vi "Fiber Auto Collimation Apex.vi"() -> ()   [LabVIEW 2018]
doc: "This is the actual top-level VI. It is called \"Apex\" instead of \"Main\" because it has the command handling in it but it's not the main front panel, so it's not a \"Main\" VI in the usual sense."
uses:
  State data/Permission levels.ctl
  <userlib>/Recipe/Station Config/Station config.lvclass
  C:/Program Files (x86)/National Instruments/LabVIEW 2018/user.lib/Recipe/nLight Recipe/nLight Recipe.lvclass
  State data/Fiber Auto Collimation state data.lvclass
  Panels/Fiber Auto Collimation panel.lvclass
  <instrlib>/nLight Instruments/Beam Profiler/Beam Profiler.lvclass
  <instrlib>/nLight Instruments/Motion Controller/Specific Models/Thorlabs Kinesis/Thorlabs motion.lvclass
  <instrlib>/nLight Instruments/Motion Controller/Motion Controller.lvclass
  <instrlib>/nLight Instruments/Motion Controller/Specific Models/Thorlabs Kinesis/Monitor/Thorlabs Monitor.lvclass
  <userlib>/nEQdb/Test Data classes/Test Data.lvclass
  <userlib>/nEQdb/Test Data classes/Standard Laser Data/Standard Laser Data.lvclass
  C:/Program Files (x86)/National Instruments/LabVIEW 2018/user.lib/nEQdb/Test Data classes/Test Data.lvclass
  <instrlib>/nLight Instruments/Beam Profiler/Specific Models/BeamView/BeamView.lvclass
  State data/Fiber Auto Collimation state data.lvclass/Fiber Auto Collimation state data.ctl
  State data/Station status.ctl
  State data/String keys.ctl
  <userlib>/Recipe/Station Config/Station config.lvclass/Station config.ctl
  <instrlib>/nLight Instruments/nLight Instrument/nLight Instrument.lvclass
  <userlib>/nLight Tidbits/Logging/Controls/Logging type choice.ctl
  Error handling/Model error handling data.ctl
  Queueing/Model queue data.ctl
  <userlib>/Recipe/nLight Recipe/Recipe problem handling method.ctl
  <userlib>/Recipe/WebService/Base URI for MOM recipe management.ctl
  Queueing/Selective queue clearing methods.ctl
  <userlib>/nLight Tidbits/Logging/Controls/Logging setup FGV options.ctl
  <userlib>/nLight Tidbits/Logging/Controls/Logging to options.ctl
  State data/Tracked state data.ctl
  <userlib>/Recipe/Station Config/Bulk startup options.ctl
  State data/Instrument list.ctl
  Panels/Main panel/Fiber Auto Collimation main panel.lvclass
  <instrlib>/nLight Instruments/Motion Controller/Axis index.ctl
  Panels/Configuration panel/Fiber Auto Collimation configuration panel.lvclass
  C:/LabVIEW Code/Fiber Auto Collimation/Source/Panels/Fiber Auto Collimation panel.lvclass
  State data/Boolean keys.ctl
  State data/Integer keys.ctl
  State data/Float keys.ctl
  <userlib>/Recipe/Test Recipe classes/Test Recipe.lvclass
  c91f844a-f770-4daa-9f60-3301e0a5f322.vi
  b3d8b4fd-21fb-468c-bd3f-db48a488eb2a.vi
  efb2ec2a-33ad-4281-ad92-67e4d6b6ec68.vi
  ae384ee7-eaaf-47a0-aaff-5ccb6f93d8a1.vi
  a18a64c1-f4c2-4f15-aef6-8607d0dc9e34.vi
  997a605e-7b1f-4adb-a0e7-d1eb57c4fb87.vi
  c0a0718e-5dff-4a87-91f2-0d7809bf613b.vi
  82acb594-edb5-4f8a-8fca-e4c401c4994d.vi
  54d7c561-c5ff-4c4f-ad18-53407e4e607b.vi
  2cd3d775-6c45-4b39-8171-6f7e11c70f95.vi
  8a1b4983-7c71-4597-b233-a9b8e1038a8c.vi
  eb02f1ea-705f-4cce-9035-a9f8b34ca533.vi
  828f032b-9937-4802-b0e2-0a19cdc0ac1c.vi
  76d71b13-37a6-4cc4-9b9a-5e2ce6ce3de4.vi
  d3521ccb-280c-4964-8afe-59c39be19f88.vi
  12af3aa9-4c13-45d6-86bd-f229a8c437ee.vi
  <userlib>/nLight Tidbits/Misc/Convert True to Enabled.vi
  997a605e-7b1f-4adb-a0e7-d1eb57c4fb87.vi/a2caca50-23ab-4663-8cbd-eebdf5a4aabe.vi
  c0a0718e-5dff-4a87-91f2-0d7809bf613b.vi/9db3fc61-2e1c-4885-9405-90c6bc597e16.vi
  References/Obtain control updates queue.vi
  Misc SubVIs/Get control name.vi
  <vilib>/Utility/Data Type/Get Type Information.vi
  <userlib>/nLight Error Handling/Log any errors.vi
  <userlib>/nLight Error Handling/Replace string to enum conversion error.vi
  <vilib>/Platform/browser.llb/Open URL in Default Browser (string).vi
  <userlib>/nLight Error Handling/Replace class conversion error.vi
  <instrlib>/nLight Instruments/Motion Controller/Move axis relative static wrapper.vi
  <userlib>/Recipe/nLight Recipe/nLight Recipe.lvclass
  <userlib>/Recipe/Station Setup/Station setup.lvclass
  <userlib>/nEQdb/Test Data classes/Test Setup Data/Test Setup data.lvclass
  96201640-59f3-40c7-bccc-0d3a8a55a5b1.vi
  <instrlib>/nLight Instruments/Monitor/Monitor.lvclass
  438d002f-1f4e-4f37-9de9-ab7f762d22aa.vi
  References/Fiber Auto Collimation References.lvclass
panel:
  out "Station status":string
  out "Permission level":T1
  out "Username":string
  out "Currently running state":string
  in  "Upload station config":bool
  in  "Configure instruments":bool
  in  "Edit station config keys":bool
  in  "Basic station config":bool
  out "Station information":string="Software name: \nSoftware version:\nSite: \nEnvironment: \nNEQdb Station number: \nMOM Equipment ID: "
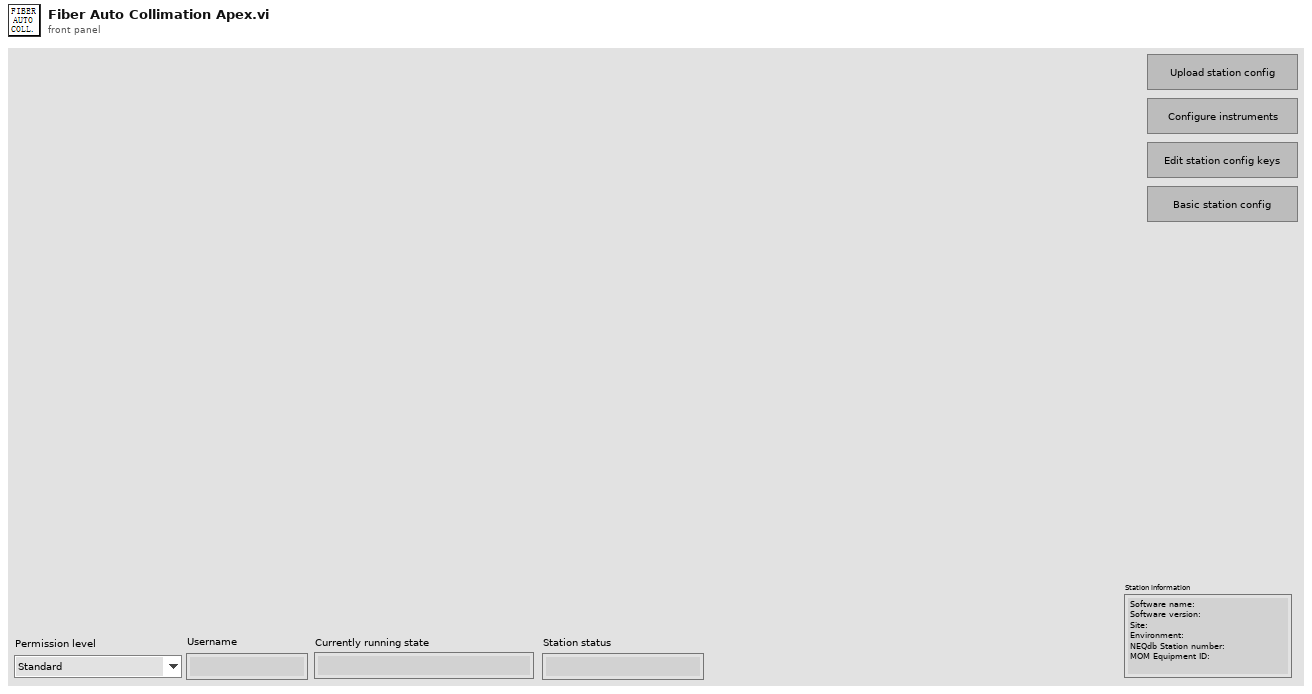
[diagram p1: front panel]
types:
  T1 = typedef "Fiber Auto Collimation state data.lvclass/Permission levels.ctl" = enum16{"Standard", "Technician", "Engineer"}
  T2 = cluster{"事件注册引用句柄":refnum<event-registration>, "事件注册引用句柄":refnum<event-registration>}
  T3 = typedef "Fiber Auto Collimation state data.lvclass/Station status.ctl" = enum16{"Start-up, no config", "Start-up, config loaded", "Start-up, config problem", "Running", "Shutting down"}
  T4 = typedef "Logging type choice.ctl" = enum16{"No log type selected", "Testing start/stop", "Test progress", "Station startup/shutdown", "Station config change", "Recipe load/change", "Inventory transaction", "Instrument", "Debug"}
  T5 = typedef "Model error handling data.ctl" = cluster{"Removed queue elements":T6[], "Error to handle":errorcluster, "Originating state":string}
  T6 = typedef "Model queue data.ctl" = cluster{"State":string, "Data":variant, "Next state if error":string}
  T7 = typedef "Base URI for MOM recipe management.ctl" = enum16{"Default Production", "Vancouver Production", "Vancouver Test", "Hillsboro Production", "Hillsboro Test", "Shanghai Production", "Shanghai Test", "Development", "Localhost"}
  T8 = typedef "nLight Recipe.lvclass/Recipe problem handling method.ctl" = enum16{"Clear problems", "Check for problems, make no errors", "Convert problems to errors"}
  T9 = typedef "Fiber Auto Collimation state data.lvclass/String keys.ctl" = enum16{"Software version", "Software name", "Collimation Steps Data Path", "Collimation Data Path", "Defect detection Image Path"}
  T10 = typedef "Selective queue clearing methods.ctl" = enum16{"Clear entire queue", "Clear all that match", "Clear all that don't match", "Clear one of each match"}
  T11 = typedef "Fiber Auto Collimation state data.lvclass/Tracked state data.ctl" = enum16{"No update", "Permission level", "Username", "Test running", "DUT Serial", "Test status", "MOM Lot", "Loaded test recipe", "Model case running", "Station status", "BV data", "Defect Identify data", "Axis Position data", "Fiber Ass PN", "Operator", "RunTime", "VBAI", "Steps Cycle Time"}
  T12 = typedef "Logging to options.ctl" = enum16{"No selection made", "Log to file", "Log to event log", "Log to file and event log", "Log internally only"}
  T13 = typedef "Logging setup FGV options.ctl" = enum16{"Get logging options", "Set logging options", "Disable all logging", "Enable logging"}
  T14 = typedef "Station config.lvclass/Bulk startup options.ctl" = enum16{"Do nothing", "Initialize all", "Initialize for station startup", "Initialize DUT(s) only", "Initialize for test"}
  T15 = typedef "Fiber Auto Collimation state data.lvclass/Instrument list.ctl" = enum16{""}
  T16 = typedef "Motion Controller.lvclass/Axis index.ctl" = i32
  T17 = typedef "IMAQ Image.ctl" = refnum<image>
  T18 = typedef "VBAIInterface.ctl" = refnum<k21>
  T19 = typedef "Fiber Auto Collimation state data.lvclass/Float keys.ctl" = enum16{"Start position", "Peak Resp min", "Circularity min", "Beam Size Target", "Beam Size Percentage", "Stop position"}
  T20 = typedef "Fiber Auto Collimation state data.lvclass/Integer keys.ctl" = enum16{""}
  T21 = typedef "Fiber Auto Collimation state data.lvclass/Boolean keys.ctl" = enum16{"Save Collimation Steps Data Enable", "Defect detection Enable"}
  T22 = typedef "nLight Recipe.lvclass/Key name and type.ctl" = cluster{"Key name":string, "Key type":T23}
  T23 = typedef "nLight Recipe.lvclass/Key pair types.ctl" = enum16{"None", "Float", "Integer", "String", "Boolean"}
  T24 = typedef "MOMiCommon.ctl" = cluster{"ApplicationName":string, "ScreenName":string, "EmpNum":string, "Langauge":string}
  T25 = typedef "Standard Laser Data.lvclass/Subtest index.ctl" = cluster{"Index":i32}
  T26 = typedef "Standard Laser Data.lvclass/Data point index.ctl" = cluster{"Index":i32}
  T27 = typedef "LIV data set.ctl" = cluster{"Slope efficiency":dbl[unit], "Threshold current":dbl[unit], "LIV test data":T28[], "Meas temperature":dbl[unit], "Test start":string, "Test finish":string, "Set temperature":dbl[unit], "Voltage intercept":dbl[unit], "Resistance":dbl[unit], "Power auxilary units":string, "Power auxilary description":string, "Temperature auxilary description":string, "ITAR":bool, "Nominal operating power":dbl[unit], "Temperature auxilary 2 description":string, "PowerCorrectionFactor":dbl, "OpticalPwrMeterMultiplier":dbl, "OpticalPwrMeterOffset":dbl, "FFS Ch":u32}
  T28 = typedef "LIV datapoint.ctl" = cluster{"Set current":sgl[unit], "Measured current":sgl[unit], "Diode voltage":sgl[unit], "Compliance voltage":sgl[unit], "Optical power":sgl[unit], "Efficiency (%)":sgl, "Measured temperature":dbl[unit], "Aux power":sgl[unit], "TEC current":sgl[unit], "TEC voltage":sgl[unit], "Detector responsivity wavelength":sgl[unit], "Detector responsivity":sgl[unit], "Auxilary temperature":sgl[unit], "ITAR":bool, "Auxilary temperature 2":sgl[unit], "INTERNAL_OPTICAL_POWER:":sgl[unit], "OPTICAL_DUTY_FACTOR":sgl, "AMBIENT_GAIN_PHOTODIODE":sgl[unit], "AMBIENT_PHOTODIODE_1":sgl[unit], "AMBIENT_PHOTODIODE_2":sgl[unit], "BEAM_DUMP_PHOTODIODE":sgl[unit], "CLAD_LIGHT_STRIPPER_PHOTODIODE_1A":sgl[unit], "CLAD_LIGHT_STRIPPER_PHOTODIODE_1B":sgl[unit], "CLAD_LIGHT_STRIPPER_PHOTODIODE_2A":sgl[unit], "CLAD_LIGHT_STRIPPER_PHOTODIODE_2B":sgl[unit], "COMBINER_IN_PHOTODIODE":sgl[unit], "COMBINER_OUT_PHOTODIODE_1":sgl[unit], "COMBINER_OUT_PHOTODIODE_2":sgl[unit], "FIBER_TRAY_PHOTODIODE":sgl[unit], "MANDREL_PHOTODIODE":sgl[unit], "SPLICE_PHOTODIODE_1":sgl[unit], "SPLICE_PHOTODIODE_2":sgl[unit], "AMBIENT_TEMPERATURE_1":sgl[unit], "AMBIENT_TEMPERATURE_2":sgl[unit], "BEAM_DUMP_TEMPERATURE":sgl[unit], "CLAD_LIGHT_STRIPPER_TEMPERATURE":sgl[unit], "CLAD_LIGHT_STRIPPER_TEMPERATURE_1":sgl[unit], "CLAD_LIGHT_STRIPPER_TEMPERATURE_2":sgl[unit], "CLAD_LIGHT_STRIPPER_TEMPERATURE_3":sgl[unit], "COMBINER_TEMPERATURE_1":sgl[unit], "COMBINER_TEMPERATURE_2":sgl[unit], "LDD_TEMPERATURE_1":sgl[unit], "LDD_TEMPERATURE_2":sgl[unit], "LDD_TEMPERATURE_3":sgl[unit], "LDD_TEMPERATURE_4":sgl[unit], "LDD_TEMPERATURE_5":sgl[unit], "LDD_TEMPERATURE_6":sgl[unit], "LDD_TEMPERATURE_7":sgl[unit], "DEW_POINT_TEMPERATURE":sgl[unit], "WATER_TEMPERATURE_SUPPLY":sgl[unit], "WATER_TEMPERATURE_RETURN":sgl[unit], "LDD1_VDC":sgl[unit], "LDD2_VDC":sgl[unit], "LDD3_VDC":sgl[unit], "LDD4_VDC":sgl[unit], "LDD5_VDC":sgl[unit], "LDD6_VDC":sgl[unit], "WATER_LEAK":sgl[unit], "FAN_TACH_1":sgl[unit], "FAN_TACH_2":sgl[unit], "FAN_TACH_3":sgl[unit], "FAN_TACH_4":sgl[unit], "FAN_TACH_5":sgl[unit], "FAN_TACH_6":sgl[unit], "FAN_TACH_7":sgl[unit], "FAN_TACH_8":sgl[unit], "FAN_TACH_9":sgl[unit], "HUMIDITY":sgl, "PowerCorrectionFactor":sgl, "PowerOffesetFactor":sgl[unit], "Pyrometer current":sgl[unit], "Reflectometer current":sgl[unit], "LDD7_VDC":sgl[unit], "Reported Power":sgl[unit], "Raw Detector Reading ":dbl[unit], "StationPowerFactor":dbl, "StationPowerOffset":dbl[unit], "DetectorPowerFactor":dbl, "DetectorPowerOffset":dbl[unit], "Cold Plate Temperature ":dbl[unit], "Package Temperature":dbl[unit], "AOUT1":sgl[unit], "AOUT2":sgl[unit], "AOUT3":sgl[unit], "AOUT4":sgl[unit], "Real_AC_Power":dbl[unit], "AC_Power_Factor":dbl, "AC_Voltage_L1-L2":dbl[unit], "AC_Voltage_L2-L3":dbl[unit], "AC_Voltage_L3-L1":dbl[unit], "AC_Line_Current _Total":dbl[unit], "AC_Line1_Current":dbl[unit], "AC_Line2_Current":dbl[unit], "AC_Line3_Current":dbl[unit], "BaselineCorrectionFactor":dbl, "BaselineCorrectionOffset":dbl[unit], "BlastShieldFactor":dbl, "BlastShieldOffset":dbl[unit], "Fiber Clamp Temperature":dbl[unit], "Low Power Optical Feedback":dbl[unit], "CoronaMotorIndex":dbl, "CoronaMotorCount":dbl, "Analog Power Control Set":sgl[unit], "Analog Power Control Measured":sgl[unit], "FF_TH":dbl[unit], "FF_PD":sgl[unit], "Zeros":dbl, "Pump_TH":dbl[unit], "Spare1_PD":sgl[unit], "Spare1_TH":dbl[unit], "Spare2_TH":dbl[unit], "Spare3_TH":dbl[unit], "Optical_Monitor_PD":sgl[unit], "Temp1_TH":dbl[unit], "Temp2_TH":dbl[unit], "Temp3_TH":dbl[unit], "Temp4_TH":dbl[unit], "Temp5_TH":dbl[unit], "Temp6_TH":dbl[unit], "DCVolts1_VDC":sgl[unit], "DCVolts2_VDC":sgl[unit], "DCVolts3_VDC":sgl[unit], "DCVolts4_VDC":sgl[unit], "DCVolts5_VDC":sgl[unit], "DCVolts6_VDC":sgl[unit], "Water_Out_TH":dbl[unit], "Comb_TH":dbl[unit], "Optical_Monitor2_PD":sgl[unit], "Water_In_TH":dbl[unit], "PS_Air_TH":dbl[unit], "AMB_Pump_PD":sgl[unit], "BPP_PD":sgl[unit], "BPP_IN_PD":sgl[unit], "PCLS_PD":sgl[unit], "AMB_Comb_PD":sgl[unit]}
  T29 = cluster{"Set current":sgl[unit], "Optical power":sgl[unit]}
  T30 = enum32{"Invalid", "Standard", "Closed", "Hidden", "Minimized", "Maximized"}
  T31 = typedef "Station config.lvclass/Station site.ctl" = enum16{"Not set", "Vancouver", "Hillsboro", "Shanghai", "Lohja"}
  T32 = typedef "Station config.lvclass/Station environment.ctl" = enum16{"Not set", "Production", "Test", "Development"}
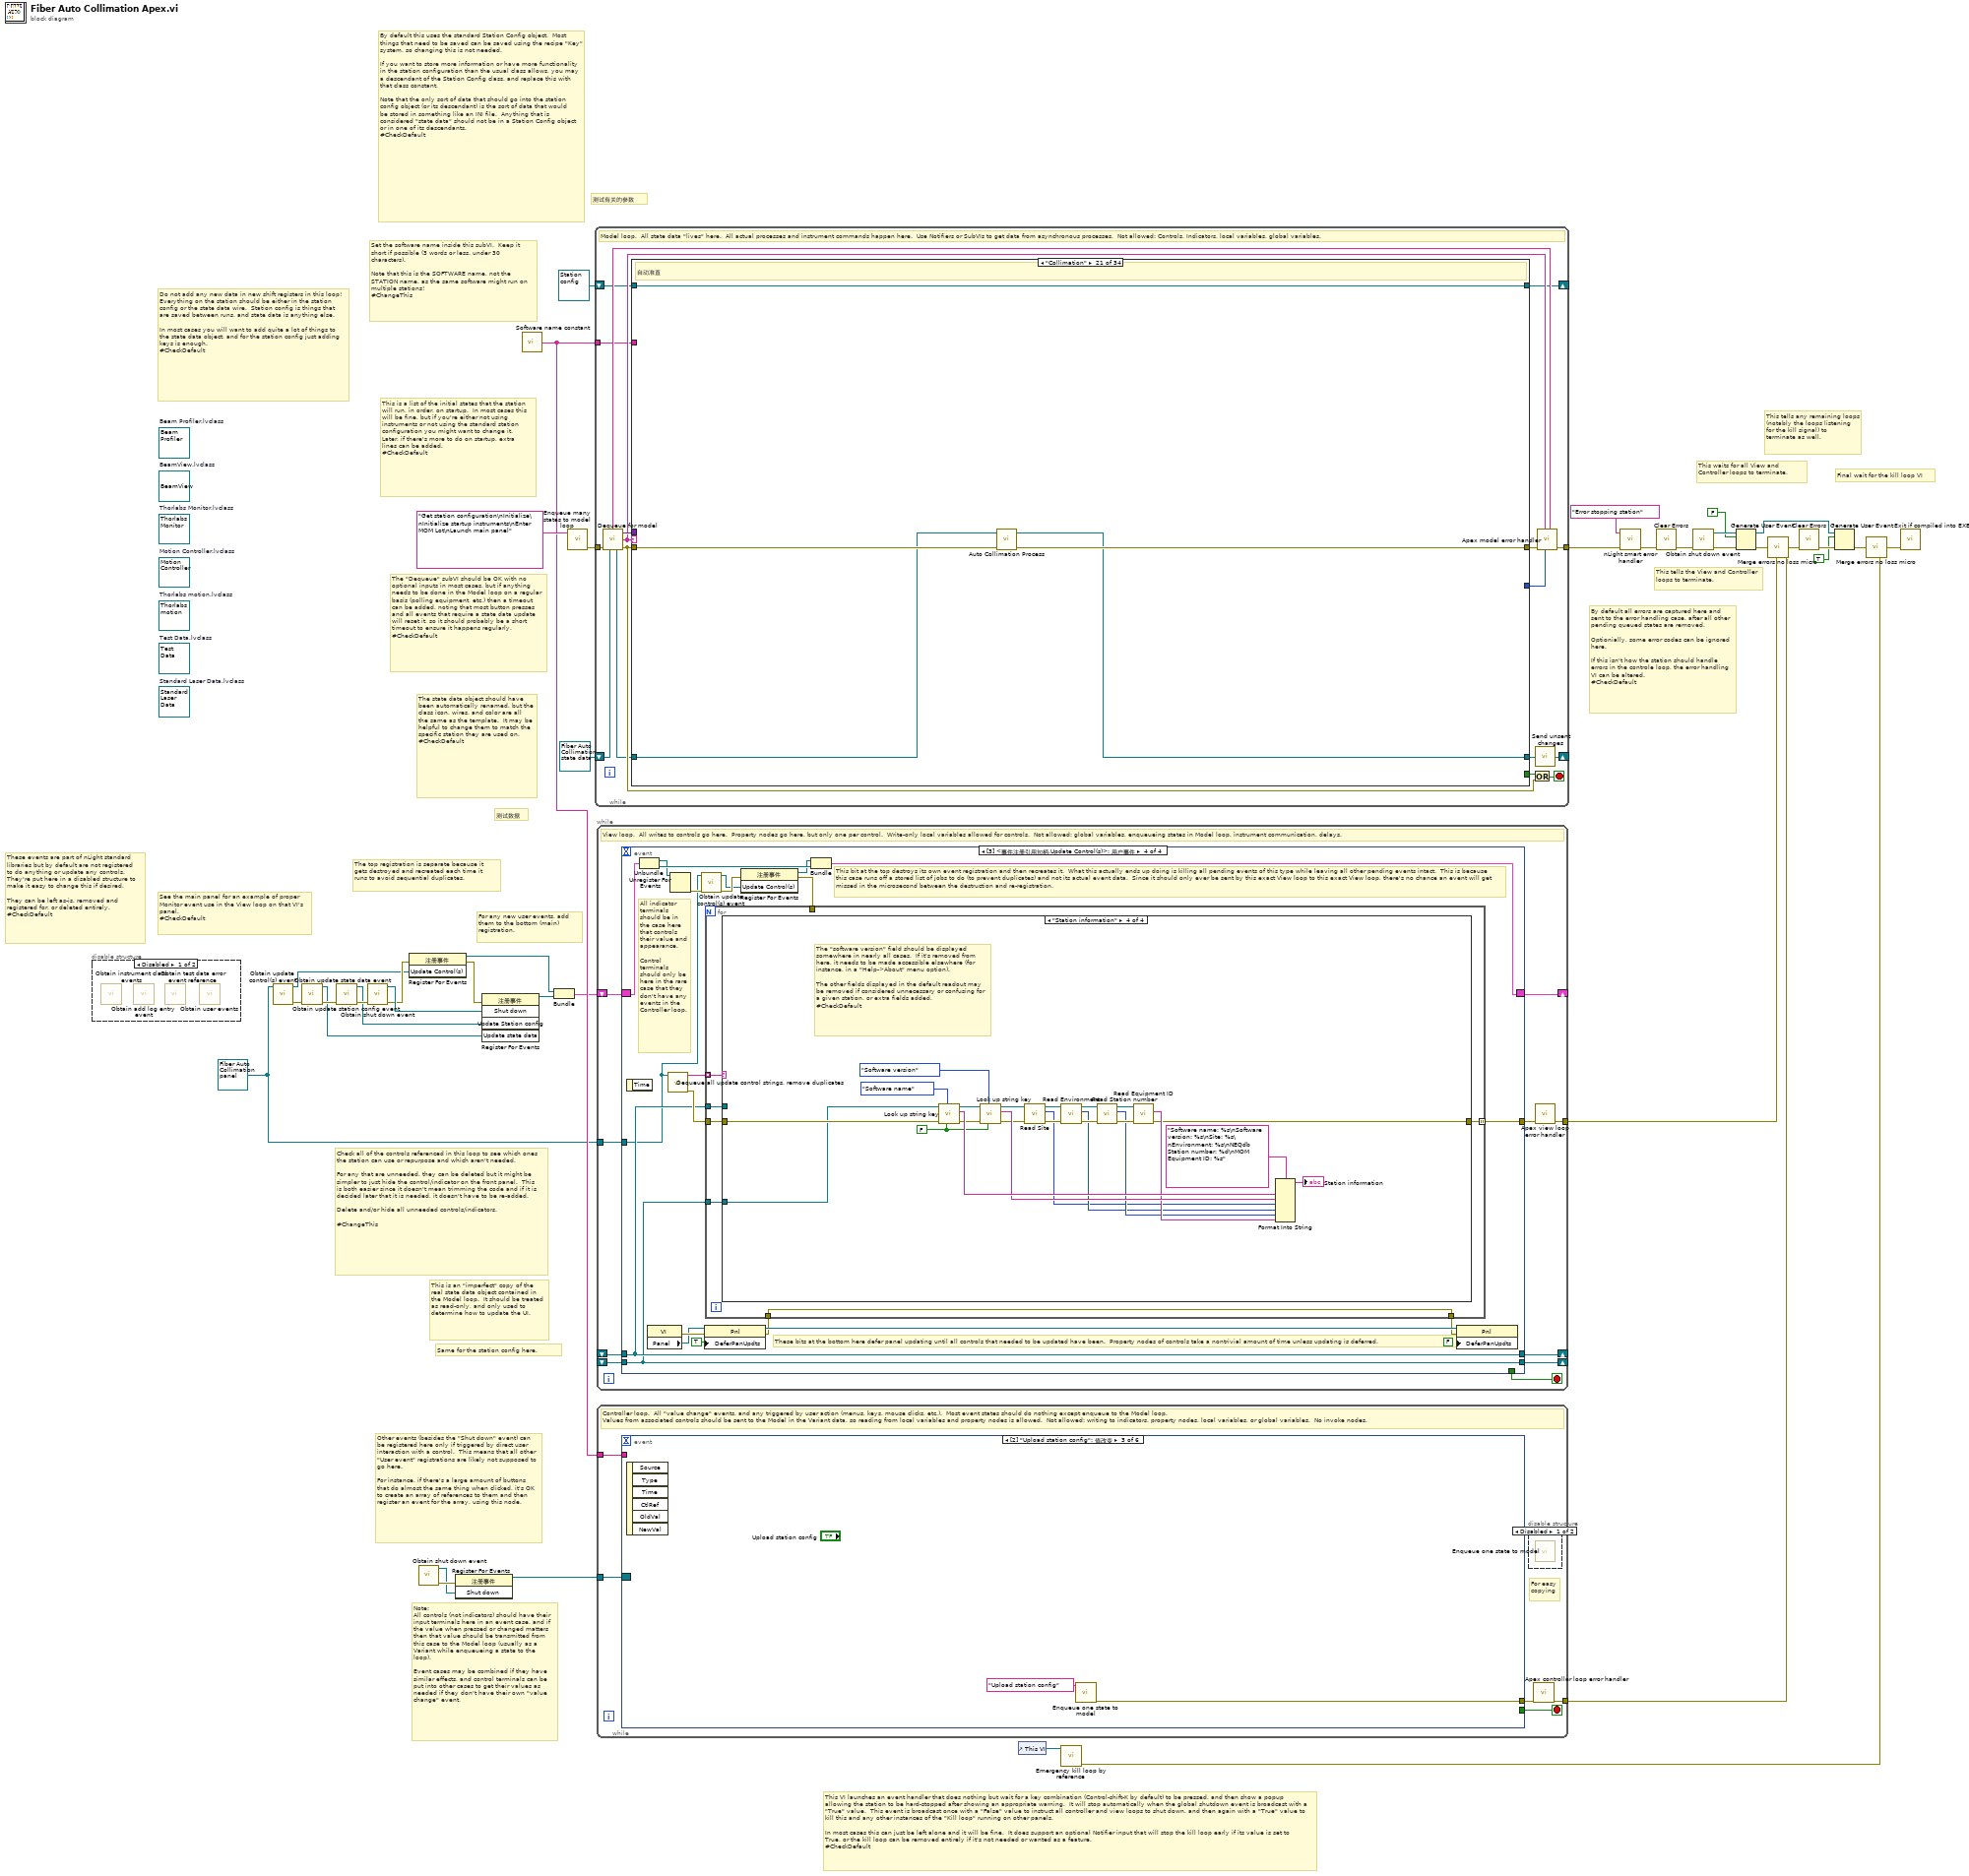
[diagram p0: block diagram]
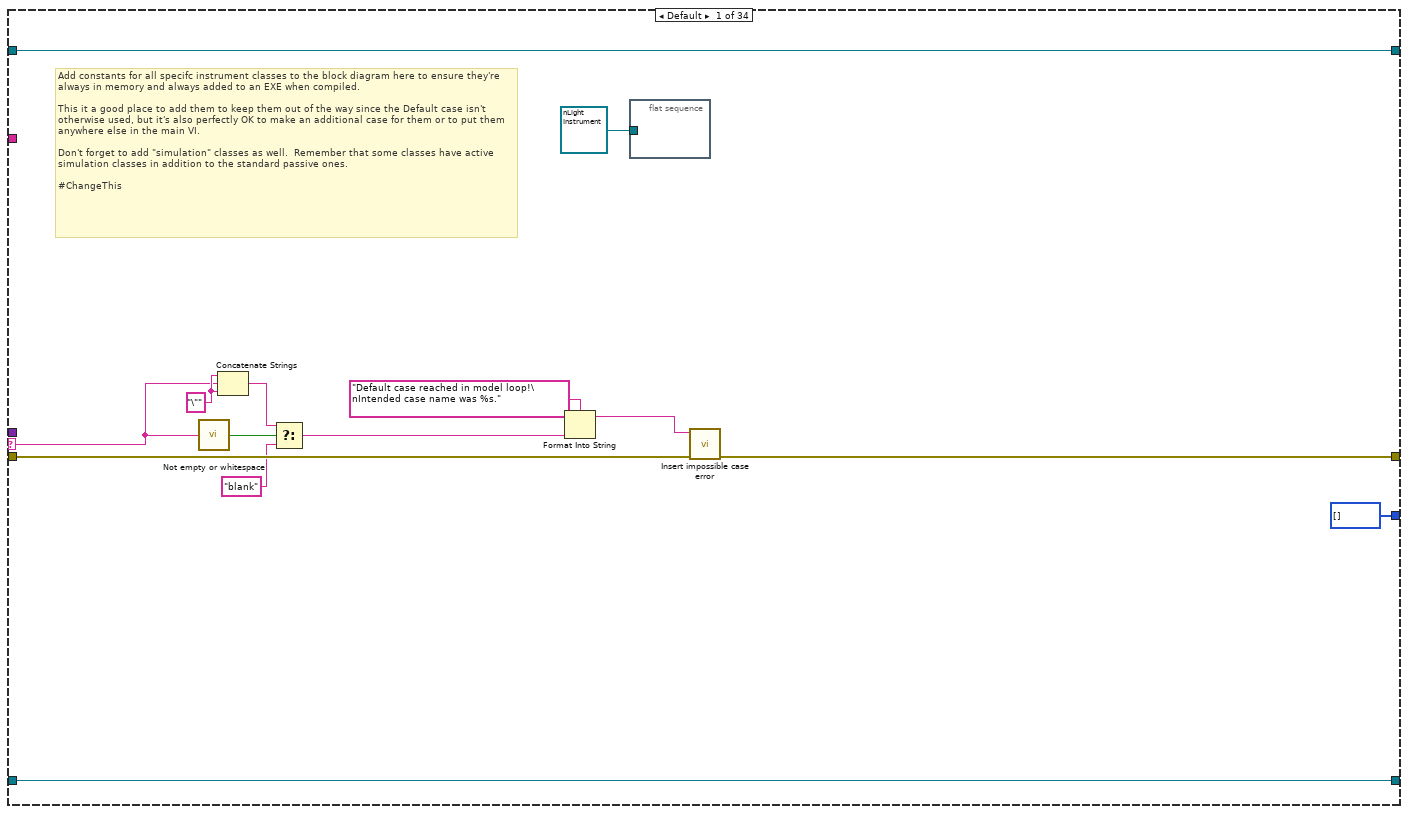
[diagram p2: hidden frame]
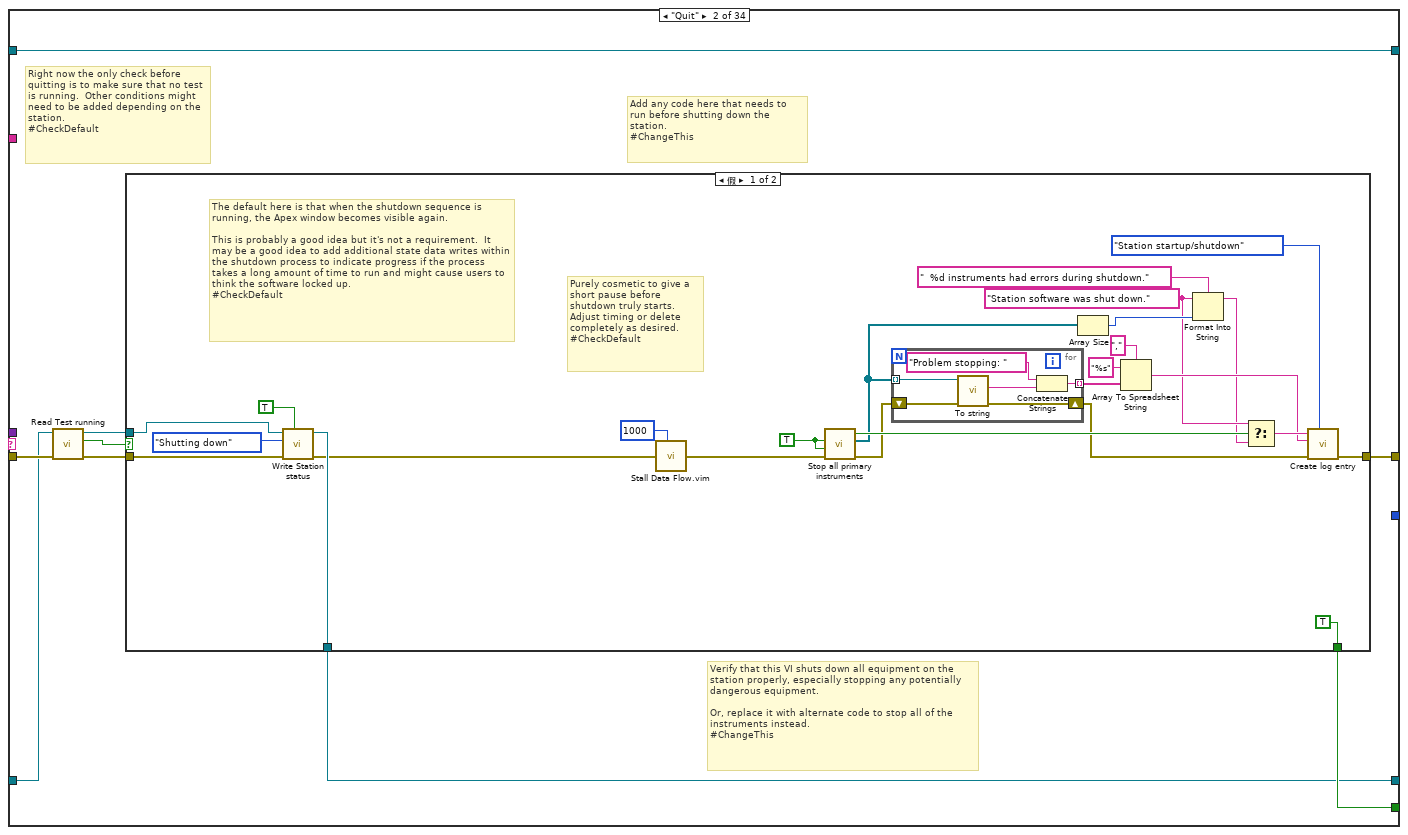
[diagram p3: hidden frame]
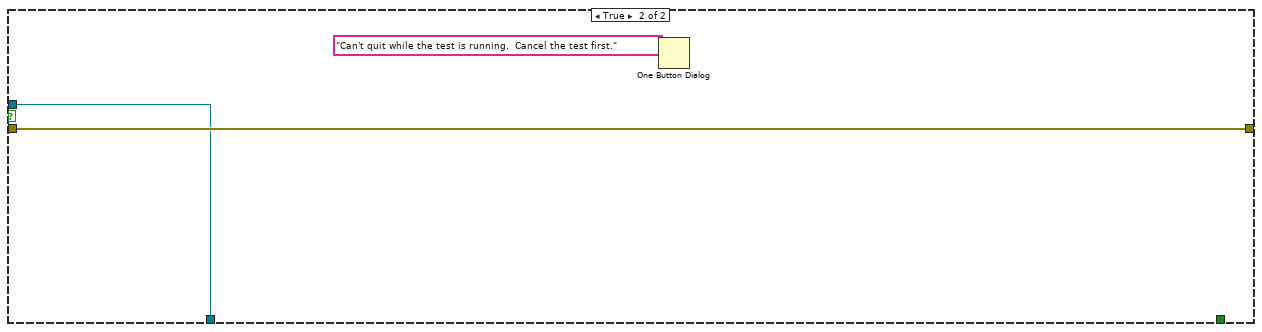
[diagram p4: hidden frame]
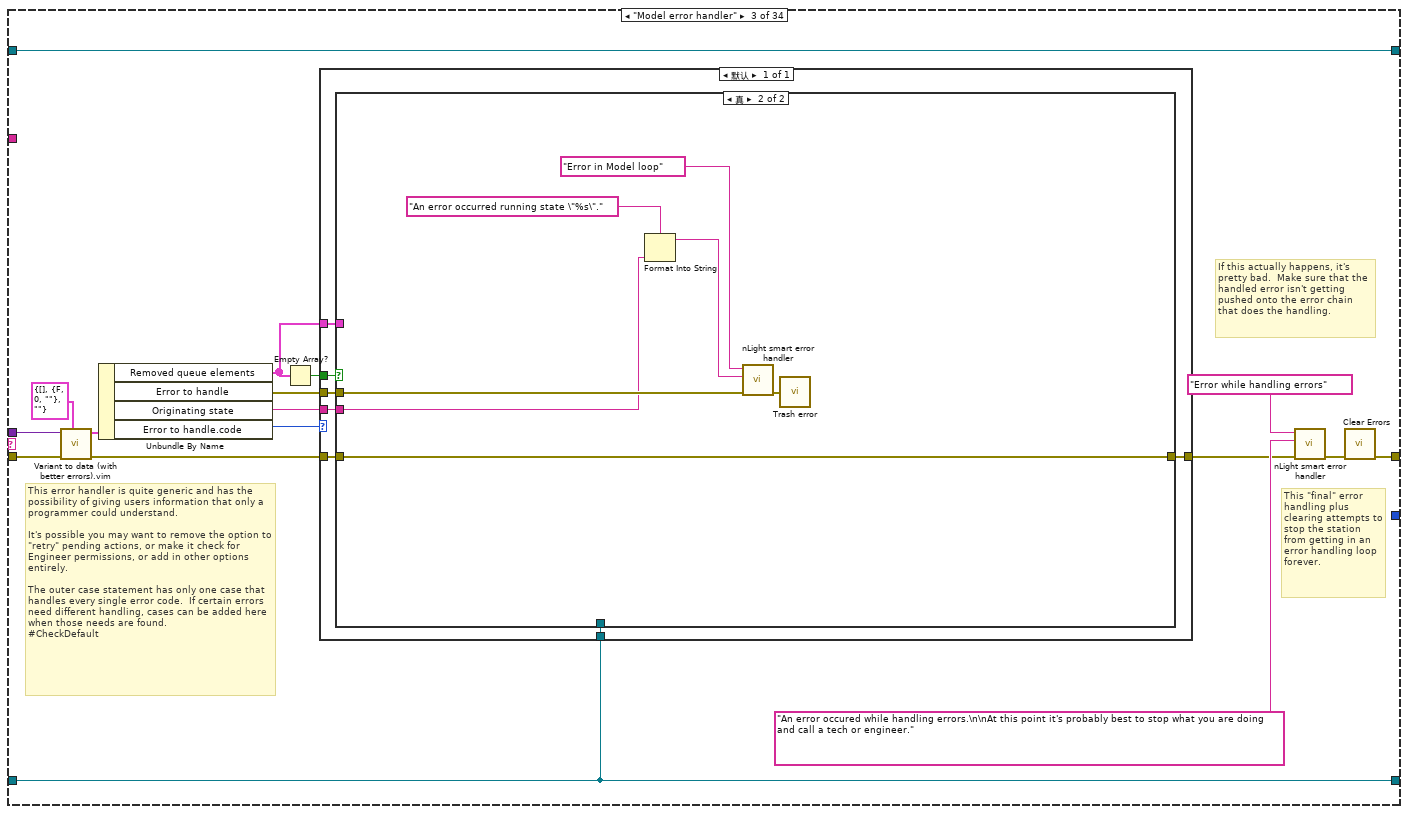
[diagram p5: hidden frame]
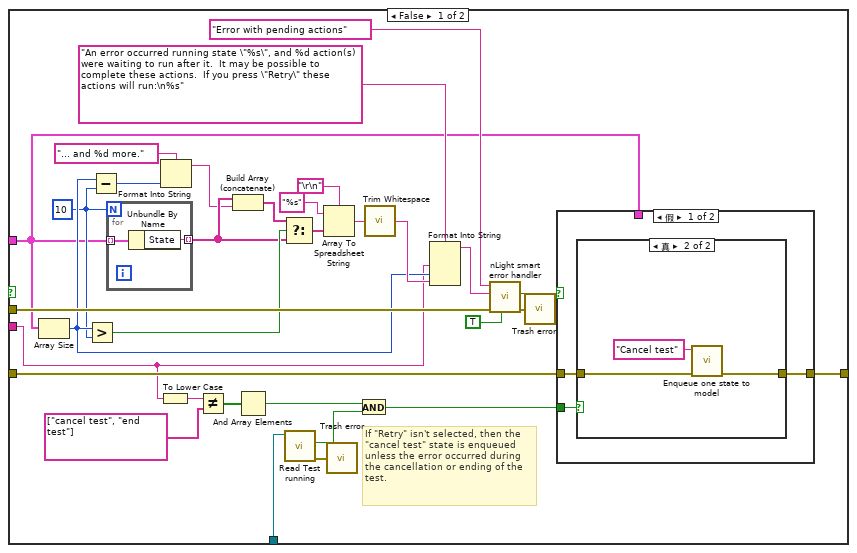
[diagram p6: hidden frame]
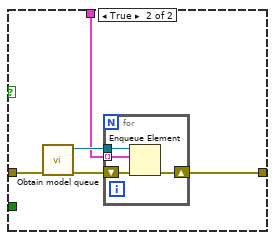
[diagram p8: hidden frame]
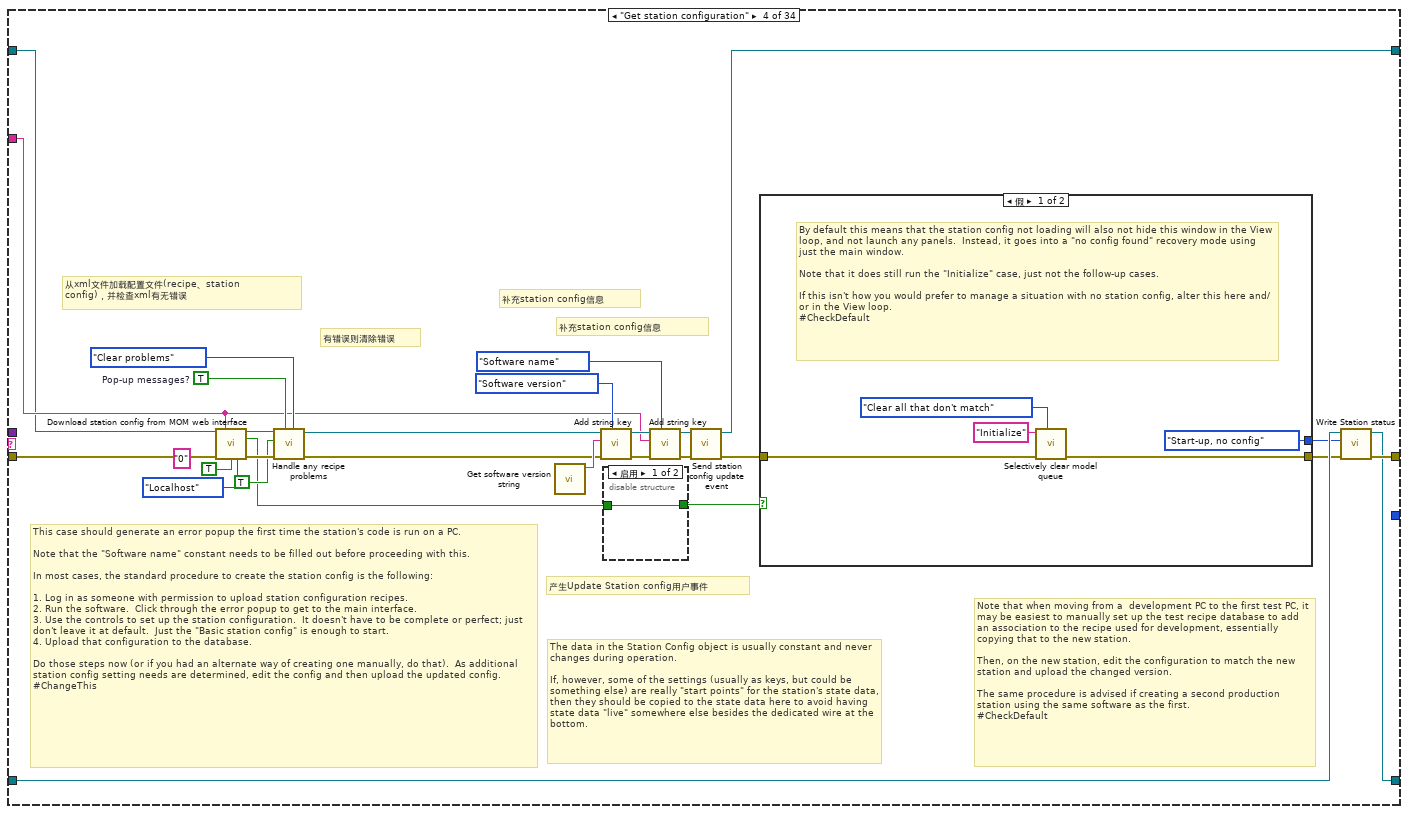
[diagram p9: hidden frame]
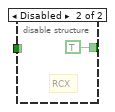
[diagram p10: hidden frame]
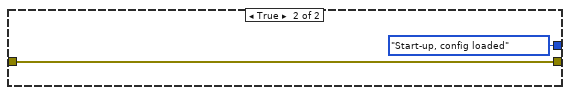
[diagram p11: hidden frame]
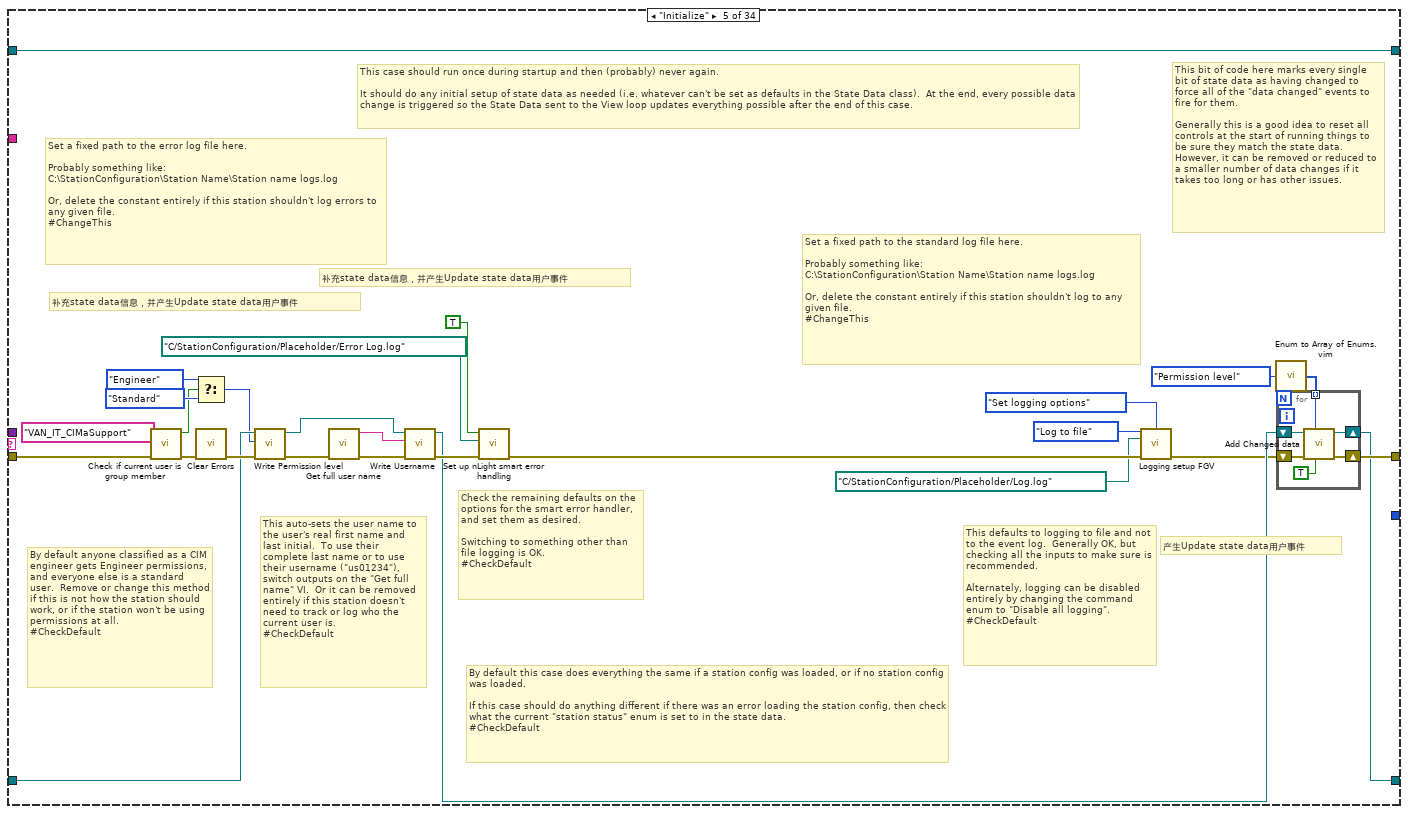
[diagram p12: hidden frame]
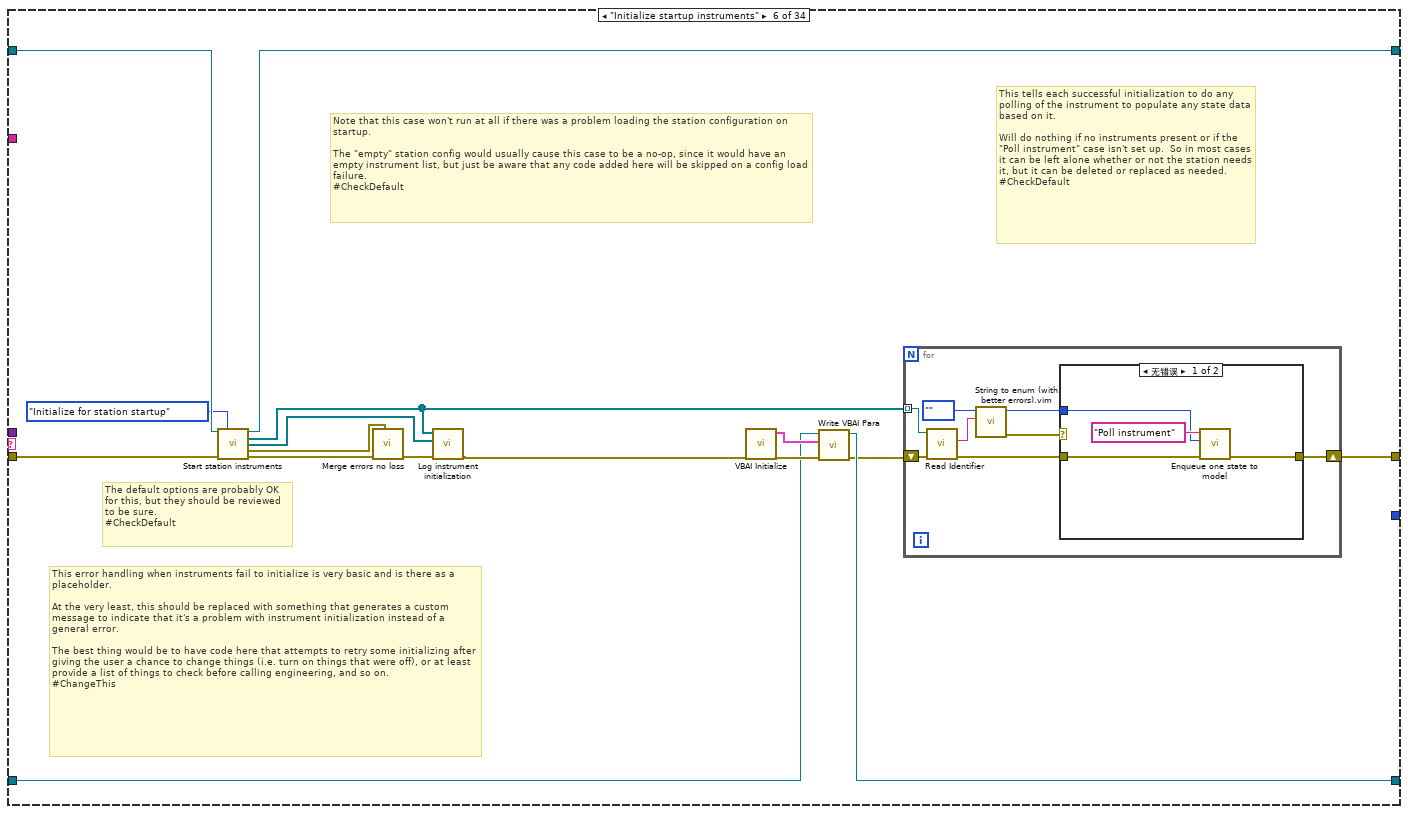
[diagram p13: hidden frame]
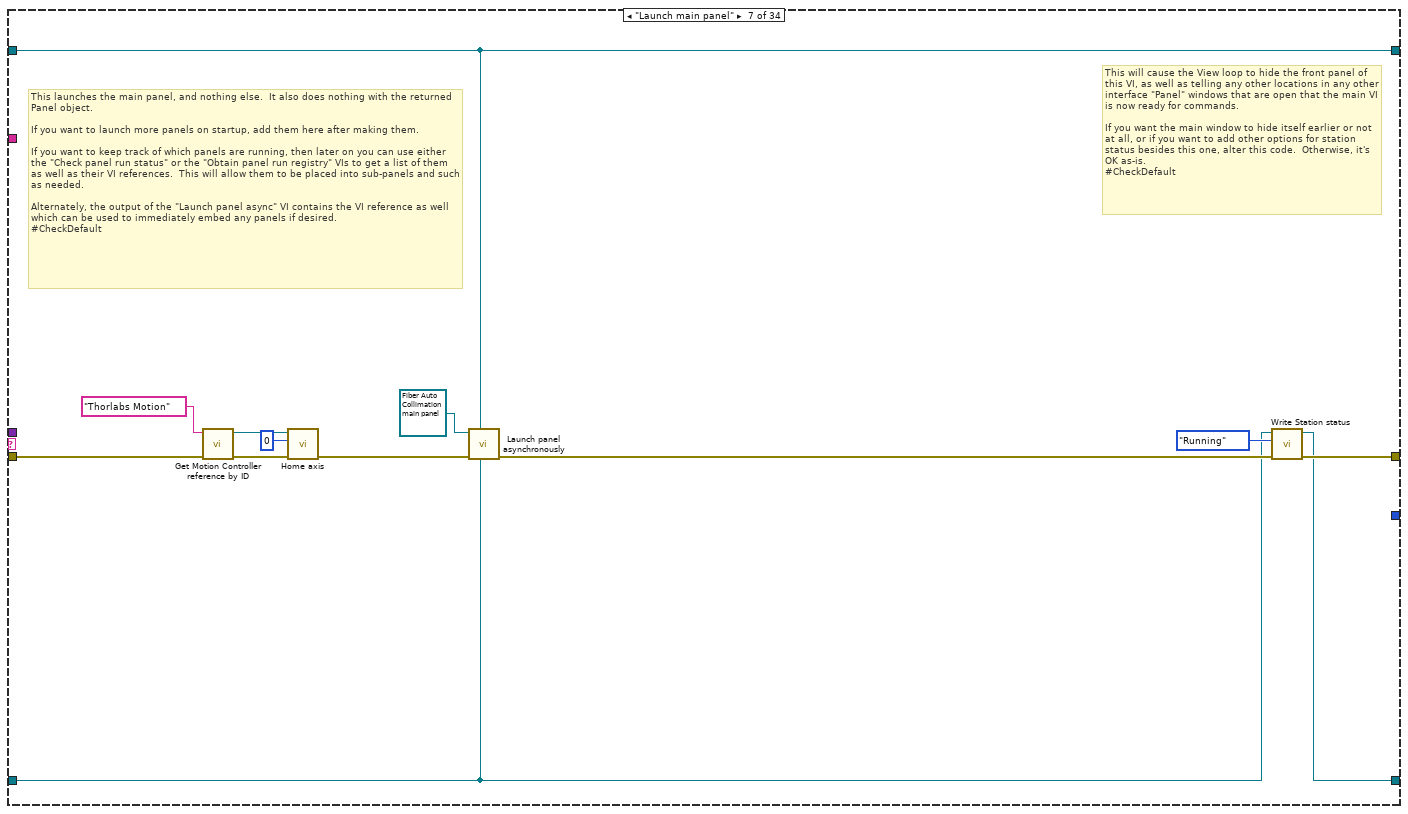
[diagram p15: hidden frame]
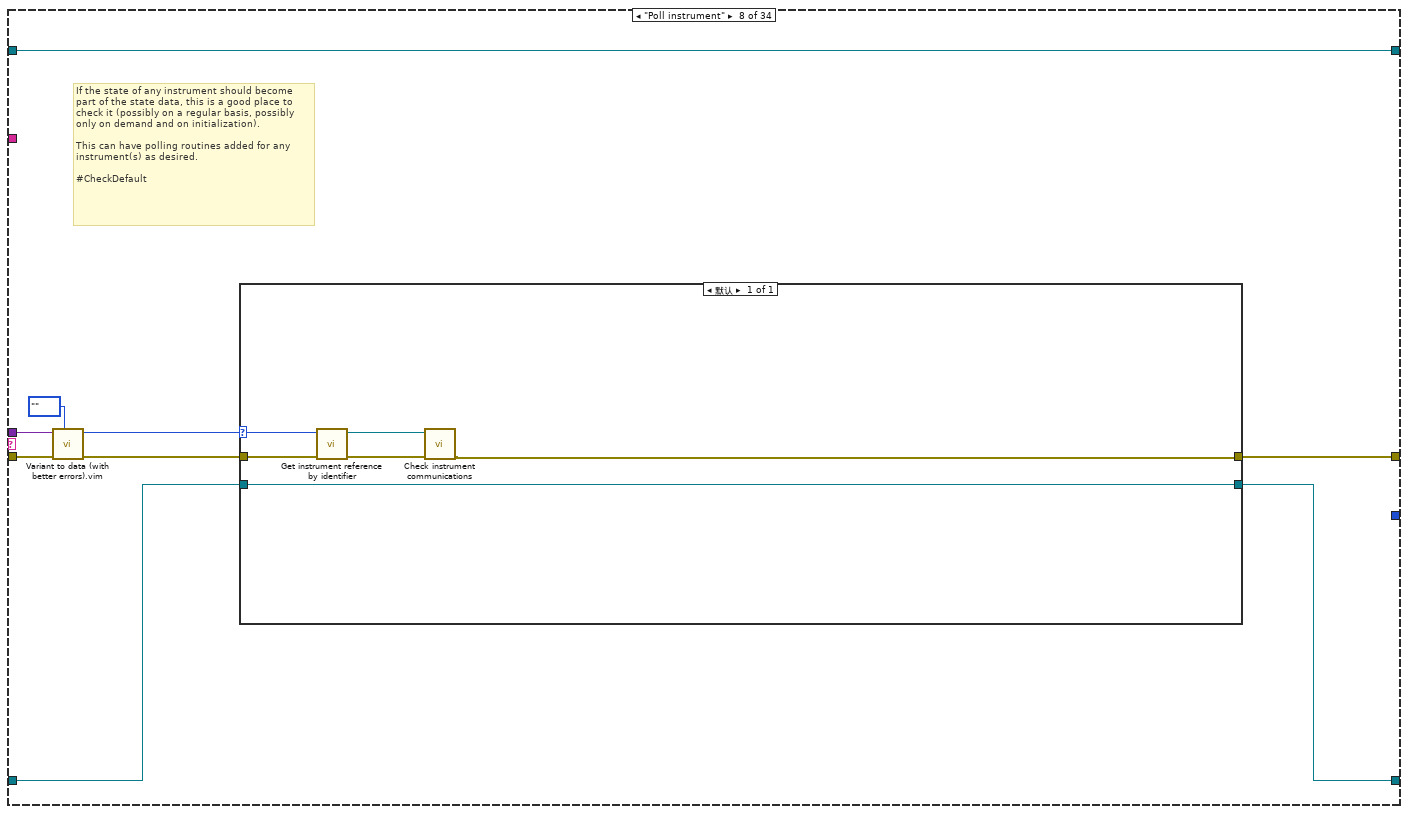
[diagram p16: hidden frame]
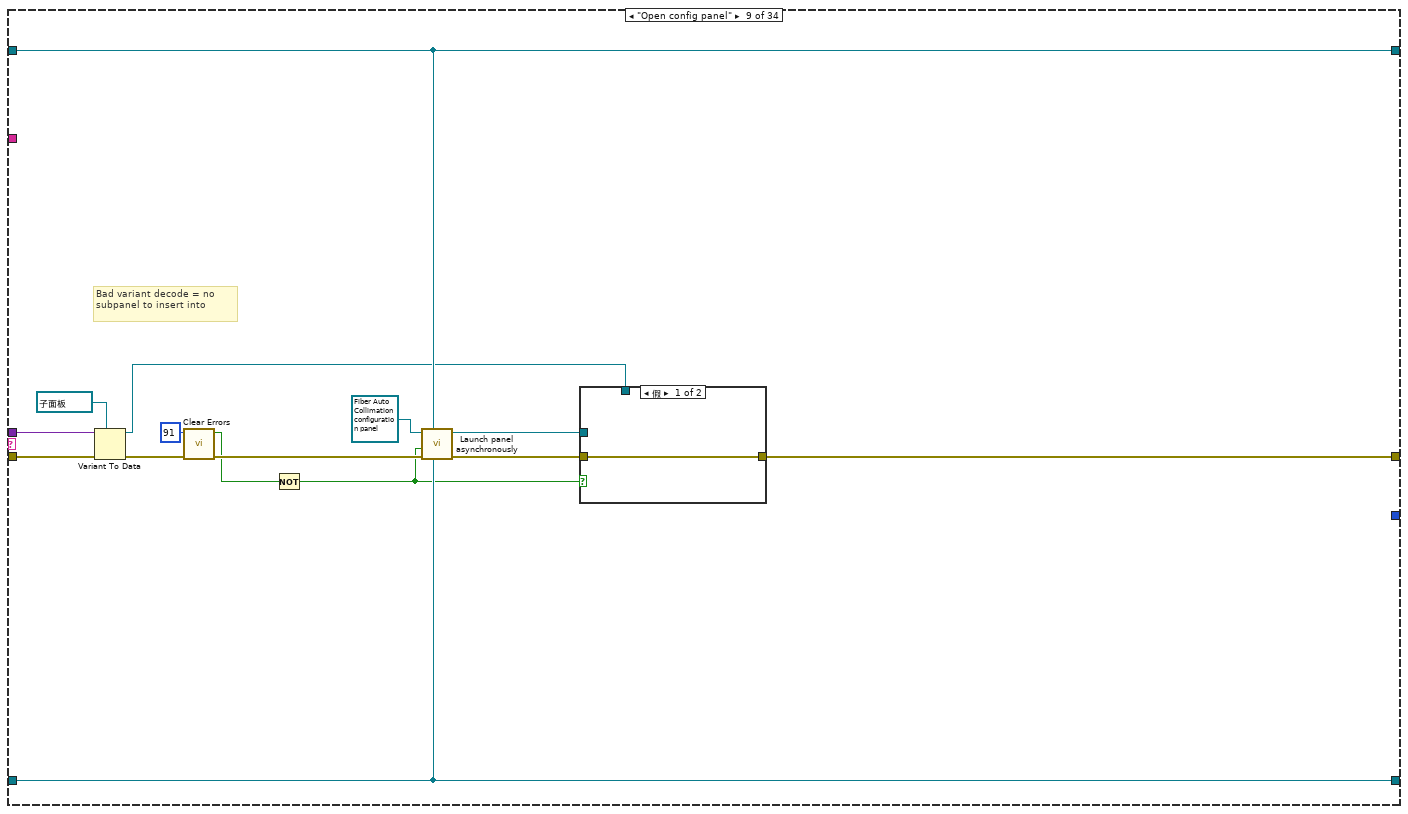
[diagram p17: hidden frame]
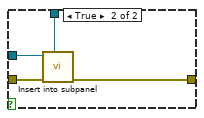
[diagram p18: hidden frame]
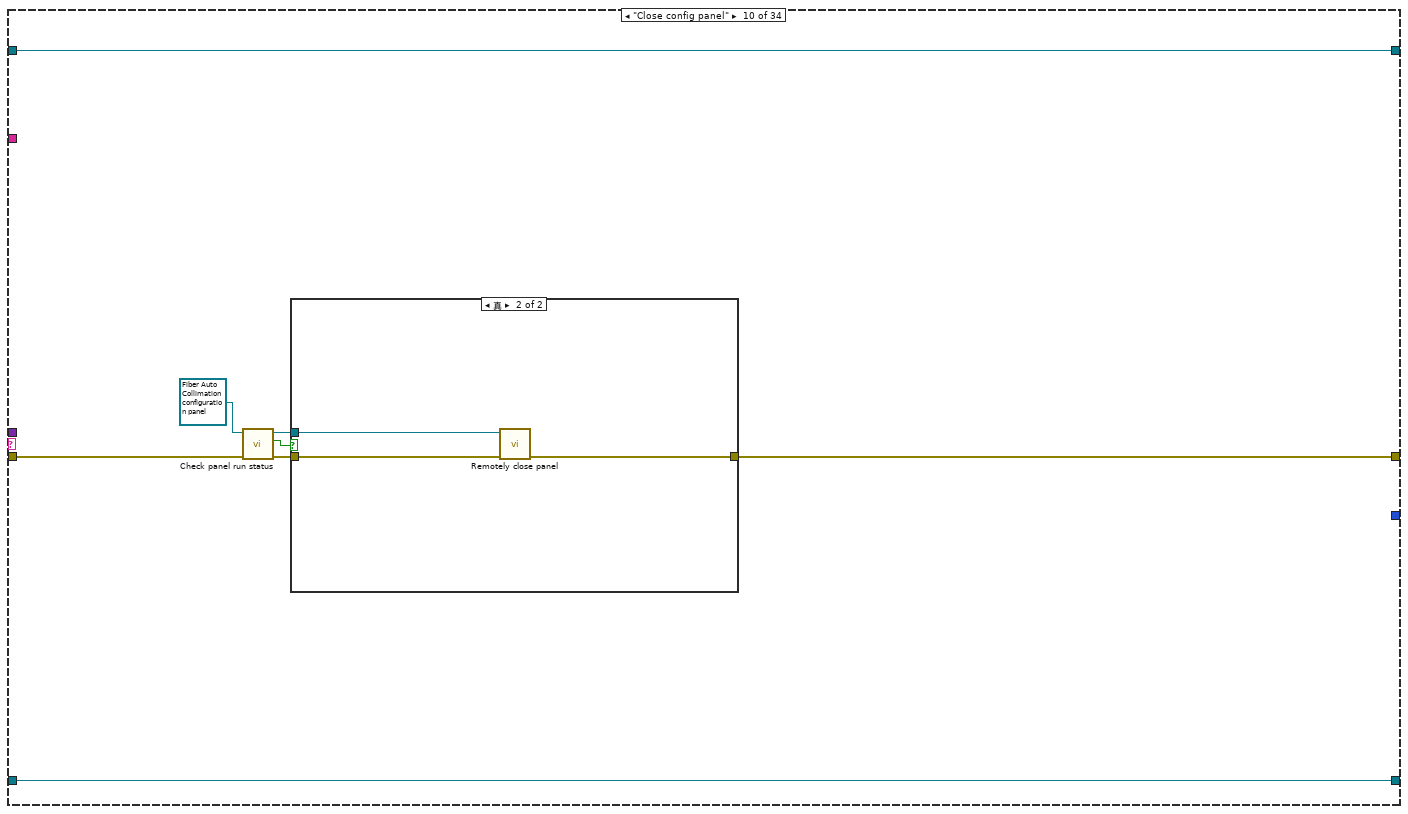
[diagram p19: hidden frame]
diagram:
  (unwired) refnum<class "BeamView.lvclass"> refnum  # BeamView.lvclass
  (unwired) refnum<class "Standard Laser Data.lvclass"> refnum  # Standard Laser Data.lvclass
  (unwired) refnum<class "Test Data.lvclass"> refnum  # Test Data.lvclass
  (unwired) refnum<class "Thorlabs Monitor.lvclass"> refnum  # Thorlabs Monitor.lvclass
  (unwired) refnum<class "Motion Controller.lvclass"> refnum  # Motion Controller.lvclass
  (unwired) refnum<class "Thorlabs motion.lvclass"> refnum  # Thorlabs motion.lvclass
  (unwired) refnum<class "Beam Profiler.lvclass"> refnum  # Beam Profiler.lvclass
  w1 = refnum<class "Fiber Auto Collimation panel.lvclass"> refnum ("Fiber Auto Collimation panel.lvclass")
  # "测试数据"
  # "测试有关的参数"
  # "This VI launches an event handler that does nothing but wait for a key combination (Control-shift-K by default) to be pressed, and then show a popup allowing the station to be hard-stopped after showing an appropriate warning.  It will stop automatically when the global shutdown event is broadcast with a \"True\" value.  This event is broadcast once with a \"False\" value to instruct all controller and view loops to shut down, and then again with a \"True\" value to kill this and any other instances of the \"Kill loop\" running on other panels.\n\nIn most cases this can just be left alone and it will be fine.  It does support an optional Notifier input that will stop the kill loop early if its value is set to True, or the kill loop can be removed entirely if it's not needed or wanted as a feature.\n#CheckDefault"
  # "Same for the station config here."
  # "See the main panel for an example of proper Monitor event use in the View loop on that VI's panel.\n#CheckDefault"
  # "Do not add any new data in new shift registers in this loop!\nEverything on the station should be either in the station config or the state data wire.  Station config is things that are saved between runs, and state data is anything else.\n\nIn most cases you will want to add quite a lot of things to the state data object, and for the station config just adding keys is enough.\n#CheckDefault"
  # "Note:\nAll controls (not indicators) should have their input terminals here in an event case, and if the value when pressed or changed matters then that value should be transmitted from this case to the Model loop (usually as a Variant while enqueueing a state to the loop).\n\nEvent cases may be combined if they have similar effects, and control terminals can be put into other cases to get their values as needed if they don't have their own \"value change\" event."
  # "Check all of the controls referenced in this loop to see which ones the station can use or repurpose and which aren't needed.  \n\nFor any that are unneeded, they can be deleted but it might be simpler to just hide the control/indicator on the front panel.  This is both easier since it doesn't mean trimming the code and if it is decided later that it is needed, it doesn't have to be re-added.\n\nDelete and/or hide all unneeded controls/indicators.\n\n#ChangeThis"
  # "Other events (besides the \"Shut down\" event) can be registered here only if triggered by direct user interaction with a control.  This means that all other \"User event\" registrations are likely not supposed to go here.\n\nFor instance, if there's a large amount of buttons that do almost the same thing when clicked, it's OK to create an array of references to them and then register an event for the array, using this node."
  # "For any new user events, add them to the bottom (main) registration."
  # "These events are part of nLight standard libraries but by default are not registered to do anything or update any controls.  They're put here in a disabled structure to make it easy to change this if desired.\n\nThey can be left as-is, removed and registered for, or deleted entirely.\n#CheckDefault"
  # "This is a list of the initial states that the station will run, in order, on startup.  In most cases this will be fine, but if you're either not using instruments or not using the standard station configuration you might want to change it.  Later, if there's more to do on startup, extra lines can be added.\n#CheckDefault"
  # "The \"Dequeue\" subVI should be OK with no optional inputs in most cases, but if anything needs to be done in the Model loop on a regular basis (polling equipment, etc.) then a timeout can be added, noting that most button presses and all events that require a state data update will reset it, so it should probably be a short timeout to ensure it happens regularly.\n#CheckDefault"
  # "The top registration is separate because it gets destroyed and recreated each time it runs to avoid sequential duplicates."
  # "The state data object should have been automatically renamed, but the class icon, wires, and color are all the same as the template.  It may be helpful to change them to match the specific station they are used on.\n#CheckDefault"
  # "By default all errors are captured here and sent to the error handling case, after all other pending queued states are removed.  \n\nOptionially, some error codes can be ignored here.\n\nIf this isn't how the station should handle errors in the controle loop, the error handling VI can be altered.\n#CheckDefault"
  # "This is an \"imperfect\" copy of the real state data object contained in the Model loop.  It should be treated as read-only, and only used to determine how to update the UI."
  # "By default this uses the standard Station Config object.  Most things that need to be saved can be saved using the recipe \"Key\" system, so changing this is not needed.\n\nIf you want to store more information or have more functionality in the station configuration than the usual class allows, you may a descendant of the Station Config class, and replace this with that class constant.\n\nNote that the only sort of data that should go into the station config object (or its descendant) is the sort of data that would be stored in something like an INI file.  Anything that is considered \"state data\" should not be in a Station Config object or in one of its descendants.\n#CheckDefault"
  # "Final wait for the kill loop VI"
  # "This tells any remaining loops (notably the loops listening for the kill signal) to terminate as well."
  # "This waits for all View and Controller loops to terminate."
  # "This tells the View and Controller loops to terminate."
  # "Set the software name inside this subVI.  Keep it short if possible (3 words or less, under 30 characters).\n\nNote that this is the SOFTWARE name, not the STATION name, as the same software might run on multiple stations!\n#ChangeThis"
  n1 = disable-structure shown="Disabled" {
    frame Disabled {
      n2 = call <instrlib>:"Obtain instrument class events.vi"() -> ()  [unwired: 7 in, 5 out]
      n3 = call <userlib>:"Obtain add log entry event.vi"() -> ()  [unwired: 10 in, 2 out]
      n4 = call <userlib>:"Obtain test data error event reference.vi"() -> ()  [unwired: 10 in, 2 out]
      n5 = call <instrlib>:"Obtain user events.vi"() -> ()  [unwired: 4 in, 8 out]
    }
    frame Enabled {
    }
  }
  n6 = call "Obtain update control(s) event.vi"("Fiber Auto Collimation panel"=w1) -> ("error out"=w9:errorcluster, "Update Control(s)"=w6:refnum<user-event>)  [unwired: 9 in]
  n7 = call "Obtain update state data event.vi"("error in (no error)"=w9) -> ("error out"=w39:errorcluster, "Update state data"=w12:refnum<user-event>)  [unwired: 9 in]
  n8 = call "Obtain update station config event.vi"("error in"=w39) -> ("error out"=w16:errorcluster, "Update Station config"=w15:refnum<user-event>)  [unwired: 9 in]
  n9 = call "Obtain shut down event.vi"("error in (no error)"=w16) -> ("error out"=w8:errorcluster, "Shut down"=w23:refnum<user-event>)  [unwired: 9 in]
  n10 = register-events(error in=w8, w6) -> (reference out=w5:refnum<event-registration>, error out=w7:errorcluster)  [unwired: 1 in]
  n11 = call "Obtain shut down event.vi"() -> ("error out"=w22:errorcluster, "Shut down"=w21:refnum<user-event>)  [unwired: 10 in]
  n12 = register-events(error in=w22, w21) -> (reference out=w20:refnum<event-registration>)  [unwired: 1 in, 1 out]
  n13 = register-events(error in=w7, w23, w15, w12) -> (reference out=w10:refnum<event-registration>)  [unwired: 1 in, 1 out]
  n14 = call "Software name constant.vi"() -> ("Software name constant"=w14:string)
  n15 = Bundle("事件注册引用句柄"=w5, "事件注册引用句柄"=w10) -> (w11:T2)  [unwired: 1 in]
  n16 = call "Enqueue many states to model loop.vi"("Enqueued states"="Get station configuration\nInitialize\nInitialize startup instruments\nEnter MOM Lot\nLaunch main panel") -> ("error out"=w19:errorcluster)  [unwired: 8 in, 2 out]
  n17 = while {
    tunnel: [w49] -> w38
    tunnel: w14 -> [w48]
    tunnel: w19 -> [w47]
    shift-right: [w46] -> _
    shift-left: refnum<class "Station config.lvclass"> refnum ("Station config out") -> [w45]
    shift-right: [w43] -> _
    shift-left: refnum<class "Fiber Auto Collimation state data.lvclass"> refnum ("Fiber Auto Collimation state data.lvclass") -> [w41]
    stop <- w53 stop-if-true
    # "Model loop.  All state data \"lives\" here.  All actual processes and instrument commands happen here.  Use Notifiers or SubVIs to get data from asynchronous processes.  Not allowed: Controls, Indicators, local variables, global variables."
    n18 = call "Dequeue for model.vi"("error in (no error)"=w47, "Fiber Auto Collimation state data in"=w41) -> ("Next state if error"=w51:string, "Data"=w56:variant, "Enqueued state"=w50:string, "Fiber Auto Collimation state data out"=w40:refnum<class "Fiber Auto Collimation state data.lvclass">, "error out"=w52:errorcluster)  [unwired: 9 in]
    n19 = case shown="\"Collimation\"" w50 {
      selector: w50 -> [w65 _ _ _ _ _ _ _ _ _ _ _ _ _ _ _ _ _ _ _ _ _ _ _ _ _ _ _ _ _ _ _ _ _]
      tunnel: w52 -> [w70 w77 w130 w223 w258 w281 w295 w315 w337 w347 w362 w391 w425 w459 w476 w516 w550 w584 w702 w762 w851 w855 w862 w867 w873 w881 w896 w918 w932 w950 w977 w985 w994 w1002]
      tunnel: w56 -> [_ _ w129 _ _ _ _ w314 w336 _ _ _ _ _ _ _ _ _ _ _ _ _ _ _ _ _ _ _ w930 w946 w975 w984 w993 w1003]
      tunnel: [w61 w78 w122 w204 w239 w272 w307 w310 w326 w343 w358 w385 w417 w454 w478 w507 w544 w580 w705 w764 w850 w854 w861 w866 w872 w884 w888 w903 w934 w947 w970 w979 w988 w997] -> w55
      tunnel: [_ w73 _ _ _ _ _ _ _ _ _ _ _ _ _ _ _ _ _ _ _ _ _ _ _ _ _ _ _ _ _ _ _ _] -> w54
      tunnel: w48 -> [_ _ _ w208 _ _ _ _ _ _ _ _ _ w457 _ _ _ _ _ _ _ _ _ _ _ _ _ _ _ _ _ _ _ _]
      tunnel: [w60 w79 w116 w205 w259 w280 w303 w316 w332 w350 w357 w386 w415 w458 w477 w517 w551 w585 w703 w765 w849 w856 w857 w863 w869 w885 w897 w920 w945 w969 w978 w987 w996 w1005] -> w46
      tunnel: w45 -> [w60 w79 w116 w207 w259 w279 w303 w316 w332 w350 w355 w380 w413 w458 w477 w517 w551 w585 w703 w765 w849 w856 w858 w863 w868 w885 w897 w920 w945 w969 w978 w987 w996 w1005]
      tunnel: w40 -> [w59 w76 w114 w202 w251 w269 w302 w309 w331 w349 w356 w384 w414 w451 w471 w515 w549 w579 w706 w761 w848 w853 w860 w865 w871 w879 w894 w906 w925 w949 w973 w981 w990 w1000]
      tunnel: [w59 w71 w114 w203 w238 w268 w306 w308 w331 w349 w356 w384 w414 w451 w472 w508 w549 w578 w704 w763 w847 w852 w859 w864 w870 w882 w895 w905 w933 w948 w974 w980 w989 w999] -> w44
      tunnel: [i32[] [] ("Error codes to ignore (none)") _ _ _ _ _ _ _ _ _ _ _ _ _ _ _ _ _ _ _ _ _ _ _ _ _ _ _ _ _ _ _ _ _] -> w42
      frame Default {
        w66 = "\""
        # "Add constants for all specifc instrument classes to the block diagram here to ensure they're always in memory and always added to an EXE when compiled.\n\nThis it a good place to add them to keep them out of the way since the Default case isn't otherwise used, but it's also perfectly OK to make an additional case for them or to put them anywhere else in the main VI.\n\nDon't forget to add \"simulation\" classes as well.  Remember that some classes have active simulation classes in addition to the standard passive ones.\n\n#ChangeThis"
        n20 = call <userlib>:"Not empty or whitespace.vi"("String"=w65) -> ("Not empty or all whitespace"=w67:bool)  [unwired: 4 in]
        n21 = Concatenate Strings(w66, w65, w66) -> (w64:string)
        n22 = Select(t=w64, s=w67, f="blank" ("t")) -> (s? t:f=w62:string)
        n23 = Format Into String(format string="Default case reached in model loop!\nIntended case name was %s.", w62) -> (resulting string=w68:string)  [unwired: 2 in, 1 out]
        n24 = flat-sequence {
          tunnel: refnum<class "nLight Instrument.lvclass"> refnum ("nLight Instrument.lvclass") -> [_]
          frame #0 {
          }
        }
        n25 = call <userlib>:"Insert impossible case error.vi"("error in (no error)"=w70, "Optional extra info"=w68) -> ("error out"=w61:errorcluster)  [unwired: 9 in]
      }
      frame "Quit" {
        # "Right now the only check before quitting is to make sure that no test is running.  Other conditions might need to be added depending on the station.\n#CheckDefault"
        # "Verify that this VI shuts down all equipment on the station properly, especially stopping any potentially dangerous equipment.\n\nOr, replace it with alternate code to stop all of the instruments instead.\n#ChangeThis"
        # "Add any code here that needs to run before shutting down the station.\n#ChangeThis"
        n26 = call "Read Test running.vi"("error in (no error)"=w77, "Fiber Auto Collimation state data in"=w76) -> ("error out"=w75:errorcluster, "Test running"=w74:bool, "Fiber Auto Collimation state data out"=w72:refnum<class "Fiber Auto Collimation state data.lvclass">)  [unwired: 6 in, 1 out]
        n27 = case shown="假" w74 {
          tunnel: w75 -> [w87 w113]
          tunnel: [w103 w113] -> w78
          tunnel: [TRUE _] -> w73
          tunnel: w72 -> [w88 w111]
          tunnel: [w85 w111] -> w71
          frame False {
            w91 = "Station software was shut down." ("initial string")
            w104 = TRUE ("Merge instrument problems with main error out? (F)")
            # "Purely cosmetic to give a short pause before shutdown truly starts.  Adjust timing or delete completely as desired.\n#CheckDefault"
            # "The default here is that when the shutdown sequence is running, the Apex window becomes visible again.\n\nThis is probably a good idea but it's not a requirement.  It may be a good idea to add additional state data writes within the shutdown process to indicate progress if the process takes a long amount of time to run and might cause users to think the software locked up.\n#CheckDefault"
            n28 = call "Write Station status.vi"("Send any changes now? (F)"=TRUE, "error in (no error)"=w87, "Station status"=Station_status."Shutting down", "Fiber Auto Collimation state data in"=w88) -> ("error out"=w84:errorcluster, "Fiber Auto Collimation state data out"=w85:refnum<class "Fiber Auto Collimation state data.lvclass">)  [unwired: 6 in]
            n29 = call "Stall Data Flow.vim"("value in"=w84, "milliseconds to wait"=u32 1000) -> ("value out"=w83:errorcluster)  [unwired: 1 out]
            n30 = call <instrlib>:"Stop all primary instruments.vi"("error in (no error)"=w83, "Create error if instruments remain afterwards? (F)"=w104, "Merge instrument problems with main error out? (F)"=w104) -> ("error out"=w81:errorcluster, "Instruments with errors stopping"=w94:refnum<class "nLight Instrument.lvclass">[], "Everything is OK?"=w101:bool)  [unwired: 4 in, 2 out]
            n31 = for {
              tunnel: w94 -> [w109] mode=indexing
              tunnel: [w107] -> w95 mode=indexing
              shift-right: [w105] -> w80
              shift-left: w81 -> [w106]
              n32 = call-dynamic "To string.vi"("error in (no error)"=w106, "nLight Instrument in"=w109) -> ("error out"=w105:errorcluster, "String"=w108:string)  [unwired: 7 in, 1 out]
              n33 = Concatenate Strings("Problem stopping: " ("string"), w108) -> (w107:string)
            }
            n34 = Array Size(array=w94) -> (size(s)=w102:i32)
            n35 = Array To Spreadsheet String(delimiter (Tab)=",", array=w95, 3:"%s" ("format string")) -> (spreadsheet string=w93:string)
            n36 = Format Into String(format string="  %d instruments had errors during shutdown." ("Brief log entry"), initial string=w91, w102) -> (resulting string=w90:string)  [unwired: 1 in, 1 out]
            n37 = Select(t=w91, s=w101, f=w90) -> (s? t:f=w99:string)
            n38 = call <userlib>:"Create log entry.vi"("Logging type choice"=Logging_type_choice."Station startup/shutdown", "error in (no error)"=w80, "Verbose log addition (none)"=w93, "Brief log entry"=w99) -> ("error out"=w103:errorcluster)  [unwired: 7 in]
          }
          frame True {
            n39 = One Button Dialog(message="Can't quit while the test is running.  Cancel the test first.") -> ()  [unwired: 1 in, 1 out]
          }
        }
      }
      frame "Model error handler" {
        # "If this actually happens, it's pretty bad.  Make sure that the handled error isn't getting pushed onto the error chain that does the handling."
        # "This error handler is quite generic and has the possibility of giving users information that only a programmer could understand.\n\nIt's possible you may want to remove the option to \"retry\" pending actions, or make it check for Engineer permissions, or add in other options entirely.\n\nThe outer case statement has only one case that handles every single error code.  If certain errors need different handling, cases can be added here when those needs are found.\n#CheckDefault"
        # "This \"final\" error handling plus clearing attempts to stop the station from getting in an error handling loop forever."
        n40 = call "Variant to data (with better errors).vim"("type"=T5 {"Removed queue elements"=[], "Error to handle"={"status"=FALSE, "code"=0, "source"=""}, "Originating state"=""} ("Error handling data cluster"), "error in"=w130, "variant"=w129) -> ("error out"=w126:errorcluster, "data"=w127:T5)  [unwired: 7 in]
        n41 = Unbundle By Name(w127) -> ("Removed queue elements"=w118:T6[], "Error to handle"=w124:errorcluster, "Originating state"=w123:string, "Error to handle.code"=w115:i32)
        n42 = Empty Array?(array=w118) -> (empty?=w125:bool)
        n43 = case shown="默认" w115 {
          tunnel: w126 -> [w137]
          tunnel: w125 -> [w136]
          tunnel: w124 -> [w135]
          tunnel: w123 -> [w134]
          tunnel: w118 -> [w133]
          tunnel: [w132] -> w117
          tunnel: w114 -> [w131]
          frame 默认 {
            n44 = case shown="真" w136 {
              tunnel: w137 -> [w152 w189]
              tunnel: w135 -> [w169 w194]
              tunnel: w134 -> [w147 w191]
              tunnel: w133 -> [w151 _]
              tunnel: [w150 w189] -> w132
              tunnel: w131 -> [w141 _]
              frame False {
                w159 = 10
                # "If \"Retry\" isn't selected, then the \"cancel test\" state is enqueued unless the error occurred during the cancellation or ending of the test."
                n45 = Array Size(array=w151) -> (size(s)=w160:i32)
                n46 = Greater?(x=w160, y=w159) -> (0:w165:bool)
                n47 = Subtract(x=w160, y=w159) -> (x-y=w158:i32)
                n48 = for {
                  N: w159 -> [_]
                  tunnel: w151 -> [w187] mode=indexing
                  tunnel: [w186] -> w156 mode=indexing
                  n49 = Unbundle By Name(w187) -> ("State"=w186:string)
                }
                n50 = To Lower Case(string=w147) -> (all lower case string=w146:string)
                n51 = Format Into String(format string="... and %d more.", w158) -> (resulting string=w155:string)  [unwired: 2 in, 1 out]
                n52 = Not Equal?(x=w146, y=string[] ["cancel test", "end test"] ("format string")) -> (x != y?=w144:bool[])
                n53 = Build Array (concatenate)(w156, w155) -> (w154:string[])
                n54 = And Array Elements(Boolean array=w144) -> (logical AND=w143:bool)
                n55 = Select(t=w154, s=w165, f=w156) -> (s? t:f=w164:string[])
                n56 = call "Read Test running.vi"("Fiber Auto Collimation state data in"=w141) -> ("error out"=w139:errorcluster, "Test running"=w142:bool)  [unwired: 7 in, 2 out]
                n57 = Array To Spreadsheet String(delimiter (Tab)="\r\n", array=w164, 3:"%s" ("format string")) -> (spreadsheet string=w162:string)
                n58 = call <userlib>:"Trash error.vi"("error in"=w139) -> ()  [unwired: 15 in]
                n59 = And(x=w143, y=w142) -> (x .and. y?=w140:bool)
                n60 = call <vilib>:"Trim Whitespace.vi"("string"=w162) -> ("trimmed string"=w161:string)  [unwired: 1 in]
                n61 = Format Into String(format string="An error occurred running state \"%s\", and %d action(s) were waiting to run after it.  It may be possible to complete these actions.  If you press \"Retry\" these actions will run:\n%s", w147, w160, w161) -> (resulting string=w167:string)  [unwired: 2 in, 1 out]
                n62 = call <userlib>:"nLight smart error handler.vi"("Enable \"Retry\" option (F)"=TRUE ("Enable \"Retry\" option (F)"), "error in (no error)"=w169, "Popup message if not in table (Generic message)"=w167, "Error title if not in table [<40 chars] (\"LabVIEW error\")"="Error with pending actions" ("Title [~40 chars max] (\"LabVIEW error\")")) -> ("error out"=w138:errorcluster, "\"Retry\" selected?"=w153:bool)  [unwired: 5 in, 1 out]
                n63 = call <userlib>:"Trash error.vi"("error in"=w138) -> ()  [unwired: 15 in]
                n64 = case shown="假" w153 {
                  tunnel: w152 -> [w171 w181]
                  tunnel: w151 -> [_ w178]
                  tunnel: [w170 w177] -> w150
                  tunnel: w140 -> [w172 _]
                  frame False {
                    n65 = case shown="真" w172 {
                      tunnel: w171 -> [w173 w176]
                      tunnel: [w173 w175] -> w170
                      frame False {
                      }
                      frame True {
                        n66 = call "Enqueue one state to model.vi"("error in (no error)"=w176, "Enqueued state"="Cancel test") -> ("error out"=w175:errorcluster)  [unwired: 9 in]
                      }
                    }
                  }
                  frame True {
                    n67 = call "Obtain model queue.vi"("error in (no error)"=w181) -> ("error out"=w180:errorcluster, "Model loop queue"=w179:refnum<queue>)  [unwired: 9 in]
                    n68 = for {
                      tunnel: w179 -> [w184]
                      tunnel: w178 -> [w183] mode=indexing
                      shift-right: [w182] -> w177
                      shift-left: w180 -> [w185]
                      n69 = Enqueue Element(queue=w184, element=w183, error in (no error)=w185) -> (error out=w182:errorcluster)  [unwired: 1 in, 2 out]
                    }
                  }
                }
              }
              frame True {
                n70 = Format Into String(format string="An error occurred running state \"%s\".", w191) -> (resulting string=w190:string)  [unwired: 2 in, 1 out]
                n71 = call <userlib>:"nLight smart error handler.vi"("error in (no error)"=w194, "Popup message if not in table (Generic message)"=w190, "Error title if not in table [<40 chars] (\"LabVIEW error\")"="Error in Model loop" ("Title [~40 chars max] (\"LabVIEW error\")")) -> ("error out"=w188:errorcluster)  [unwired: 6 in, 2 out]
                n72 = call <userlib>:"Trash error.vi"("error in"=w188) -> ()  [unwired: 15 in]
              }
            }
          }
        }
        n73 = call <userlib>:"nLight smart error handler.vi"("error in (no error)"=w117, "Popup message if not in table (Generic message)"="An error occured while handling errors.\n\nAt this point it's probably best to stop what you are doing and call a tech or engineer." ("Popup message (Generic message)"), "Error title if not in table [<40 chars] (\"LabVIEW error\")"="Error while handling errors" ("Title [~40 chars max] (\"LabVIEW error\")")) -> ("error out"=w121:errorcluster)  [unwired: 6 in, 2 out]
        n74 = call <vilib>:"Clear Errors.vi"("error in (no error)"=w121) -> ("error out"=w122:errorcluster)  [unwired: 5 in, 1 out]
      }
      frame "Get station configuration" {
        w213 = TRUE  # Pop-up messages?
        # "产生Update Station config用户事件"
        # "补充station config信息"
        # "补充station config信息"
        # "有错误则清除错误"
        # "从xml文件加载配置文件(recipe、station config)，并检查xml有无错误"
        # "The data in the Station Config object is usually constant and never changes during operation.\n\nIf, however, some of the settings (usually as keys, but could be something else) are really \"start points\" for the station's state data, then they should be copied to the state data here to avoid having state data \"live\" somewhere else besides the dedicated wire at the bottom."
        # "Note that when moving from a  development PC to the first test PC, it may be easiest to manually set up the test recipe database to add an association to the recipe used for development, essentially copying that to the new station.  \n\nThen, on the new station, edit the configuration to match the new station and upload the changed version.\n\nThe same procedure is advised if creating a second production station using the same software as the first.\n#CheckDefault"
        # "This case should generate an error popup the first time the station's code is run on a PC.\n\nNote that the \"Software name\" constant needs to be filled out before proceeding with this.\n\nIn most cases, the standard procedure to create the station config is the following:\n\n1. Log in as someone with permission to upload station configuration recipes.\n2. Run the software.  Click through the error popup to get to the main interface.\n3. Use the controls to set up the station configuration.  It doesn't have to be complete or perfect; just don't leave it at default.  Just the \"Basic station config\" is enough to start.\n4. Upload that configuration to the database.\n\nDo those steps now (or if you had an alternate way of creating one manually, do that).  As additional station config setting needs are determined, edit the config and then upload the updated config.  \n#ChangeThis"
        n75 = call <userlib>:"Download station config from MOM web interface.vi"("Station config model in (defaults)"=w207, "Program name"=w208, "Version (\"0\")"="0" ("Version (\"0\")"), "error in (no error)"=w223, "Show \"downloading\" message? (F)"=TRUE ("Show \"downloading\" message? (F)"), "Recipe server to use? (Default production)"=Base_URI_for_MOM_recipe_management."Localhost") -> ("Station config out"=w214:refnum<class "Station config.lvclass">, "Everything is OK?"=w197:bool, "error out"=w216:errorcluster)  [unwired: 4 in, 3 out]
        n76 = call-dynamic "Handle any recipe problems.vi"("Recipe problem handling method"=Recipe_problem_handling_method."Clear problems", "Pop-up messages?"=w213, "error in (no error)"=w216, "Can override problems? (F)"=TRUE, "nLight Recipe in"=w214) -> ("error out"=w215:errorcluster, "nLight Recipe out"=w209:refnum<class "Station config.lvclass">)  [unwired: 3 in, 2 out]
        n77 = call "Get software version string.vi"() -> ("Software version string"=w222:string)  [unwired: 11 in]
        n78 = call <userlib>:"Add string key.vi"("Key [string/enum]"=String_keys."Software version" ("Station config string keys"), "error in (no error)"=w215, "String value"=w222, "nLight Recipe in"=w209) -> ("error out"=w220:errorcluster, "nLight Recipe out"=w219:refnum<class "Station config.lvclass">)  [unwired: 5 in, 1 out]
        n79 = disable-structure shown="启用" {
          disable-tunnel: w197 -> [w224 _]
          disable-tunnel: [w224 TRUE ("Everything is OK?")] -> w196
          frame Enabled {
          }
          frame Disabled {
            # "RCX"
          }
        }
        n80 = call <userlib>:"Add string key.vi"("Key [string/enum]"=String_keys."Software name" ("Station config string keys"), "error in (no error)"=w220, "String value"=w208, "nLight Recipe in"=w219) -> ("error out"=w218:errorcluster, "nLight Recipe out"=w206:refnum<class "Station config.lvclass">)  [unwired: 5 in, 1 out]
        n81 = call "Send station config update event.vi"("error in (no error)"=w218, "Station config in"=w206) -> ("error out"=w200:errorcluster, "Station config out"=w205:refnum<class "Station config.lvclass">)  [unwired: 8 in]
        n82 = case shown="假" w196 {
          tunnel: [Station_status."Start-up, no config" ("Station status") Station_status."Start-up, config loaded" ("Station status")] -> w201
          tunnel: w200 -> [w228 w231]
          tunnel: [w227 w231] -> w199
          frame False {
            # "By default this means that the station config not loading will also not hide this window in the View loop, and not launch any panels.  Instead, it goes into a \"no config found\" recovery mode using just the main window.\n\nNote that it does still run the \"Initialize\" case, just not the follow-up cases.\n\nIf this isn't how you would prefer to manage a situation with no station config, alter this here and/or in the View loop.\n#CheckDefault"
            n83 = call "Selectively clear model queue.vi"("Queue clearing option"=Selective_queue_clearing_methods."Clear all that don't match", "error in (no error)"=w228, "State(s) to look for [One per line]"="Initialize") -> ("error out"=w227:errorcluster)  [unwired: 7 in, 1 out]
          }
          frame True {
          }
        }
        n84 = call "Write Station status.vi"("error in (no error)"=w199, "Station status"=w201, "Fiber Auto Collimation state data in"=w202) -> ("error out"=w204:errorcluster, "Fiber Auto Collimation state data out"=w203:refnum<class "Fiber Auto Collimation state data.lvclass">)  [unwired: 7 in]
      }
      frame "Initialize" {
        # "产生Update state data用户事件"
        # "补充state data信息，并产生Update state data用户事件"
        # "补充state data信息，并产生Update state data用户事件"
        # "By default this case does everything the same if a station config was loaded, or if no station config was loaded.  \n\nIf this case should do anything different if there was an error loading the station config, then check what the current \"station status\" enum is set to in the state data.\n#CheckDefault"
        # "This bit of code here marks every single bit of state data as having changed to force all of the \"data changed\" events to fire for them.  \n\nGenerally this is a good idea to reset all controls at the start of running things to be sure they match the state data.  However, it can be removed or reduced to a smaller number of data changes if it takes too long or has other issues."
        # "Check the remaining defaults on the options for the smart error handler, and set them as desired.  \n\nSwitching to something other than file logging is OK.\n#CheckDefault"
        # "This defaults to logging to file and not to the event log.  Generally OK, but checking all the inputs to make sure is recommended.\n\nAlternately, logging can be disabled entirely by changing the command enum to \"Disable all logging\".\n#CheckDefault"
        # "Set a fixed path to the standard log file here.\n\nProbably something like:\nC:\\StationConfiguration\\Station Name\\Station name logs.log\n\nOr, delete the constant entirely if this station shouldn't log to any given file.\n#ChangeThis"
        # "This auto-sets the user name to the user's real first name and last initial.  To use their complete last name or to use their username (\"us01234\"), switch outputs on the \"Get full name\" VI.  Or it can be removed entirely if this station doesn't need to track or log who the current user is.\n#CheckDefault"
        # "By default anyone classified as a CIM engineer gets Engineer permissions, and everyone else is a standard user.  Remove or change this method if this is not how the station should work, or if the station won't be using permissions at all.\n#CheckDefault"
        # "Set a fixed path to the error log file here.\n\nProbably something like:\nC:\\StationConfiguration\\Station Name\\Station name logs.log\n\nOr, delete the constant entirely if this station shouldn't log errors to any given file.\n#ChangeThis"
        # "This case should run once during startup and then (probably) never again.  \n\nIt should do any initial setup of state data as needed (i.e. whatever can't be set as defaults in the State Data class).  At the end, every possible data change is triggered so the State Data sent to the View loop updates everything possible after the end of this case."
        n85 = call <userlib>:"Check if current user is group member.vi"("error in (no error)"=w258, "Group name"="VAN_IT_CIMaSupport") -> ("error out"=w256:errorcluster, "Is Member Of"=w253:bool)  [unwired: 8 in]
        n86 = Select(t=Permission_levels."Engineer" ("Permission levels"), s=w253, f=Permission_levels."Standard" ("Permission levels")) -> (s? t:f=w250:T1)
        n87 = call <vilib>:"Clear Errors.vi"("error in (no error)"=w256) -> ("error out"=w252:errorcluster)  [unwired: 5 in, 1 out]
        n88 = call "Write Permission level.vi"("error in (no error)"=w252, "Permission levels"=w250, "Fiber Auto Collimation state data in"=w251) -> ("error out"=w248:errorcluster, "Fiber Auto Collimation state data out"=w249:refnum<class "Fiber Auto Collimation state data.lvclass">)  [unwired: 7 in]
        n89 = call <userlib>:"Get full user name.vi"("error in (no error)"=w248) -> ("error out"=w246:errorcluster, "First name last initial"=w247:string)  [unwired: 6 in, 3 out]
        n90 = call "Write Username.vi"("error in (no error)"=w246, "Username"=w247, "Fiber Auto Collimation state data in"=w249) -> ("error out"=w237:errorcluster, "Fiber Auto Collimation state data out"=w236:refnum<class "Fiber Auto Collimation state data.lvclass">)  [unwired: 7 in]
        n91 = call <userlib>:"Set up nLight smart error handling.vi"("error in (no error)"=w237, "Path to error log file (no log file)"=path "C:/StationConfiguration/Placeholder/Error Log.log" ("Log file path"), "Logging on? (F)"=TRUE) -> ("error out"=w245:errorcluster)  [unwired: 8 in]
        n92 = call <userlib>:"Logging setup FGV.vi"("Log to options"=Logging_to_options."Log to file", "Logging setup FGV command"=Logging_setup_FGV_options."Set logging options", "Log file path"=path "C:/StationConfiguration/Placeholder/Log.log", "error in (no error)"=w245) -> ("error out"=w235:errorcluster)  [unwired: 9 in, 2 out]
        n93 = call "Enum to Array of Enums.vim"("enum"=Tracked_state_data."Permission level" ("Data type")) -> ("array of enums"=w233:T11[])
        n94 = for {
          shift-right: [w264] -> w239
          shift-left: w235 -> [w265]
          shift-right: [w262] -> w238
          shift-left: w236 -> [w263]
          tunnel: w233 -> [w260] mode=indexing
          n95 = call "Add Changed data.vi"("Data changed?"=TRUE, "Data type"=w260, "error in (no error)"=w265, "Fiber Auto Collimation state data in"=w263) -> ("error out"=w264:errorcluster, "Fiber Auto Collimation state data out"=w262:refnum<class "Fiber Auto Collimation state data.lvclass">)  [unwired: 6 in]
        }
      }
      frame "Initialize startup instruments" {
        # "Note that this case won't run at all if there was a problem loading the station configuration on startup.\n\nThe \"empty\" station config would usually cause this case to be a no-op, since it would have an empty instrument list, but just be aware that any code added here will be skipped on a config load failure.\n#CheckDefault"
        # "This tells each successful initialization to do any polling of the instrument to populate any state data based on it.\n\nWill do nothing if no instruments present or if the \"Poll instrument\" case isn't set up.  So in most cases it can be left alone whether or not the station needs it, but it can be deleted or replaced as needed.\n#CheckDefault"
        # "This error handling when instruments fail to initialize is very basic and is there as a placeholder.\n\nAt the very least, this should be replaced with something that generates a custom message to indicate that it's a problem with instrument initialization instead of a general error.\n\nThe best thing would be to have code here that attempts to retry some initializing after giving the user a chance to change things (i.e. turn on things that were off), or at least provide a list of things to check before calling engineering, and so on.\n#ChangeThis"
        # "The default options are probably OK for this, but they should be reviewed to be sure.\n#CheckDefault"
        n96 = call-dynamic "Start station instruments.vi"("Station config in"=w279, "Start options"=Bulk_startup_options."Initialize for station startup", "error in (no error)"=w281) -> ("Station config out"=w280:refnum<class "Station config.lvclass">, "Initialized instruments"=w273:refnum<class "nLight Instrument.lvclass">[], "Instruments with errors"=w274:refnum<class "nLight Instrument.lvclass">[], "Instrument errors"=w276:errorcluster[], "error out"=w277:errorcluster)  [unwired: 7 in, 1 out]
        n97 = call <userlib>:"Merge errors no loss.vi"("Error in array"=w276, "error in 6 (no error)"=w277) -> ("error out"=w275:errorcluster)  [unwired: 9 in]
        n98 = call "Log instrument initialization.vi"("error in (no error)"=w275, "Instruments with errors"=w274, "Initialized instruments"=w273) -> ("error out"=w266:errorcluster)  [unwired: 8 in]
        n99 = call "VBAI Initialize.vi"("error in"=w266) -> ("error out"=w271:errorcluster, "VBAI"=w270:cluster{"New Image":T17, "VBAI Session Out":T18})  [unwired: 9 in]
        n100 = call "Write VBAI Para.vi"("error in (no error)"=w271, "VBAI"=w270, "Fiber Auto Collimation state data in"=w269) -> ("error out"=w267:errorcluster, "Fiber Auto Collimation state data out"=w268:refnum<class "Fiber Auto Collimation state data.lvclass">)  [unwired: 7 in]
        n101 = for {
          tunnel: w273 -> [w288] mode=indexing
          shift-right: [w282] -> w272
          shift-left: w267 -> [w289]
          n102 = call <instrlib>:"Read Identifier.vi"("error in (no error)"=w289, "nLight Instrument in"=w288) -> ("error out"=w284:errorcluster, "Identifier"=w287:string)  [unwired: 7 in, 1 out]
          n103 = call "String to enum (with better errors).vim"("Text to be converted"=w287, "Default enum value"=Instrument_list."" ("Instrument list")) -> ("error out"=w285:errorcluster, "Converted value out"=w283:T15)  [unwired: 8 in]
          n104 = case shown="无错误" w285 {
            tunnel: w284 -> [w293 w294]
            tunnel: w283 -> [w291 _]
            tunnel: [w290 w294] -> w282
            frame No Error {
              n105 = call "Enqueue one state to model.vi"("error in (no error)"=w293, "Enqueued data"=w291, "Enqueued state"="Poll instrument" ("Identifier")) -> ("error out"=w290:errorcluster)  [unwired: 8 in]
            }
            frame Error {
            }
          }
        }
      }
      frame "Launch main panel" {
        # "This launches the main panel, and nothing else.  It also does nothing with the returned Panel object.\n\nIf you want to launch more panels on startup, add them here after making them.\n\nIf you want to keep track of which panels are running, then later on you can use either the \"Check panel run status\" or the \"Obtain panel run registry\" VIs to get a list of them as well as their VI references.  This will allow them to be placed into sub-panels and such as needed.\n\nAlternately, the output of the \"Launch panel async\" VI contains the VI reference as well which can be used to immediately embed any panels if desired.\n#CheckDefault"
        # "This will cause the View loop to hide the front panel of this VI, as well as telling any other locations in any other interface \"Panel\" windows that are open that the main VI is now ready for commands.\n\nIf you want the main window to hide itself earlier or not at all, or if you want to add other options for station status besides this one, alter this code.  Otherwise, it's OK as-is.\n#CheckDefault"
        n106 = call <instrlib>:"Get Motion Controller reference by ID.vi"("error in (no error)"=w295, "Identifier"="Thorlabs Motion") -> ("error out"=w299:errorcluster, "Motion Controller out"=w298:refnum<class "Motion Controller.lvclass">)  [unwired: 8 in]
        n107 = call-dynamic "Home axis.vi"("error in (no error)"=w299, "Axis index"=T16 0, "Motion Controller in"=w298) -> ("error out"=w296:errorcluster)  [unwired: 7 in, 1 out]
        n108 = call-dynamic "Launch panel asynchronously.vi"("Fiber Auto Collimation state data"=w302, "Station config"=w303, "error in"=w296, "Fiber Auto Collimation panel in"=refnum<class "Fiber Auto Collimation main panel.lvclass"> refnum ("Fiber Auto Collimation main panel.lvclass")) -> ("error out"=w304:errorcluster)  [unwired: 6 in, 1 out]
        n109 = call "Write Station status.vi"("error in (no error)"=w304, "Station status"=Station_status."Running", "Fiber Auto Collimation state data in"=w302) -> ("error out"=w307:errorcluster, "Fiber Auto Collimation state data out"=w306:refnum<class "Fiber Auto Collimation state data.lvclass">)  [unwired: 7 in]
      }
      frame "Poll instrument" {
        # "If the state of any instrument should become part of the state data, this is a good place to check it (possibly on a regular basis, possibly only on demand and on initialization).\n\nThis can have polling routines added for any instrument(s) as desired.\n\n#CheckDefault"
        n110 = call "Variant to data (with better errors).vim"("type"=Instrument_list."" ("Instrument list"), "error in"=w315, "variant"=w314) -> ("error out"=w311:errorcluster, "data"=w312:T15)  [unwired: 7 in]
        n111 = case shown="默认" w312 {
          selector: w312 -> [w320]
          tunnel: w311 -> [w321]
          tunnel: [w317] -> w310
          tunnel: w309 -> [w322]
          tunnel: [w322] -> w308
          frame 默认 {
            n112 = call <instrlib>:"Get instrument reference by identifier.vi"("error in (no error)"=w321, "Identifier"=w320) -> ("error out"=w319:errorcluster, "nLight Instrument.lvclass"=w318:refnum<class "nLight Instrument.lvclass">)  [unwired: 7 in, 1 out]
            n113 = call-dynamic "Check instrument communications.vi"("error in (no error)"=w319, "nLight Instrument in"=w318) -> ("error out"=w317:errorcluster)  [unwired: 7 in, 2 out]
          }
        }
      }
      frame "Open config panel" {
        # "Bad variant decode = no subpanel to insert into"
        n114 = Variant To Data(error in=w337, type=refnum<vi> refnum ("Sub Panel example space"), Variant=w336) -> (data=w323:refnum<vi>, error out=w335:errorcluster)
        n115 = call <vilib>:"Clear Errors.vi"("error in (no error)"=w335, "specific error code to clear (0: all)"=91) -> ("error out"=w333:errorcluster, "specific error cleared?"=w328:bool)  [unwired: 4 in]
        n116 = Not(x=w328) -> (.not. x?=w324:bool)
        n117 = call-dynamic "Launch panel asynchronously.vi"("Fiber Auto Collimation state data"=w331, "Station config"=w332, "error in"=w333, "Start hidden? (F)"=w324, "Fiber Auto Collimation panel in"=refnum<class "Fiber Auto Collimation configuration panel.lvclass"> refnum ("Fiber Auto Collimation configuration panel.lvclass")) -> ("error out"=w329:errorcluster, "Fiber Auto Collimation panel out"=w325:refnum<class "Fiber Auto Collimation configuration panel.lvclass">)  [unwired: 5 in]
        n118 = case shown="假" w324 {
          tunnel: w329 -> [w338 w342]
          tunnel: w323 -> [_ w341]
          tunnel: [w338 w340] -> w326
          tunnel: w325 -> [_ w339]
          frame False {
          }
          frame True {
            n119 = call "Insert into subpanel.vi"("Subpanel to insert into"=w341, "error in (no error)"=w342, "Fiber Auto Collimation panel in"=w339) -> ("error out"=w340:errorcluster)  [unwired: 7 in, 1 out]
          }
        }
      }
      frame "Close config panel" {
        n120 = call "Check panel run status.vi"("error in (no error)"=w347, "Fiber Auto Collimation panel in"=refnum<class "Fiber Auto Collimation configuration panel.lvclass"> refnum ("Fiber Auto Collimation configuration panel.lvclass")) -> ("error out"=w345:errorcluster, "Panel(s) running"=w346:bool, "Fiber Auto Collimation panel out"=w344:refnum<class "Fiber Auto Collimation configuration panel.lvclass">)  [unwired: 6 in, 1 out]
        n121 = case shown="真" w346 {
          tunnel: w345 -> [w351 w354]
          tunnel: w344 -> [_ w353]
          tunnel: [w351 w352] -> w343
          frame False {
          }
          frame True {
            n122 = call "Remotely close panel.vi"("error in (no error)"=w354, "Fiber Auto Collimation panel in"=w353) -> ("error out"=w352:errorcluster)  [unwired: 8 in, 1 out]
          }
        }
      }
      frame "Basic station config" {
        n123 = call-dynamic "Manual setup of basic config.vi"("error in (no error)"=w362, "Station config in"=w355) -> ("error out"=w360:errorcluster, "Cancelled?"=w361:bool, "Station config out"=w359:refnum<class "Station config.lvclass">)  [unwired: 7 in]
        n124 = case shown="假" w361 {
          tunnel: w360 -> [w371 w378]
          tunnel: w359 -> [w367 w379]
          tunnel: [w370 w378] -> w358
          tunnel: [w363 w379] -> w357
          tunnel: w355 -> [w368 _]
          frame False {
            n125 = call "Send station config update event.vi"("error in (no error)"=w371, "Station config in"=w367) -> ("error out"=w369:errorcluster, "Station config out"=w363:refnum<class "Station config.lvclass">)  [unwired: 8 in]
            n126 = call-dynamic "Compare two recipes for differences.vi"("Baseline Recipe in"=w368, "Comparison Recipe in"=w363, "error in (no error)"=w369) -> ("Other recipe changes found"=w364:bool, "Other recipe changes verbose details"=w366:string, "error out"=w365:errorcluster)  [unwired: 2 in, 8 out]
            n127 = case shown="真" w364 {
              tunnel: [w372 w376] -> w370
              tunnel: w366 -> [_ w374]
              tunnel: w365 -> [w372 w373]
              frame False {
              }
              frame True {
                n128 = call <userlib>:"Create log entry.vi"("Logging type choice"=Logging_type_choice."Station config change", "error in (no error)"=w373, "Verbose log addition (none)"=w374, "Brief log entry"="Basic station config changed") -> ("error out"=w376:errorcluster)  [unwired: 7 in]
              }
            }
          }
          frame True {
          }
        }
      }
      frame "Edit station config keys" {
        w381 = Float_keys."Start position"  # Station config float keys
        w382 = Integer_keys.""  # Station config integer keys
        w383 = Boolean_keys."Save Collimation Steps Data Enable"  # Station config boolean keys
        w390 = String_keys."Software version"  # Station config string keys
        # "This is the default editor for generic recipes with keys.  It should work for initial setup by engineering.\n\nIf any of the keys need to hold values that are restricted in value (can't be blank, need to be between two limits, etc.) then a custom value editor or checker can be added later.  \n\nThis optional and is mostly so users who edit these after initial setup can't enter illegal values.\n#CheckDefault"
        # "Edit the type definitions of these 4 enums to add all names of data fields that need to be stored as part of the station configuration.\n\nThis can be delayed until later in the process of making the station software if it's not currently known everything that needs to be stored in the station configuration object.\n#ChangeThis"
        n129 = call <userlib>:"Key editor window.vi"("Boolean keys"=w383, "Integer keys"=w382, "String keys"=w390, "Float keys"=w381, "error in (no error)"=w391, "nLight Recipe in"=w380) -> ("error out"=w387:errorcluster, "Cancelled?"=w389:bool, "nLight Recipe out"=w388:refnum<class "Station config.lvclass">)  [unwired: 3 in]
        n130 = case shown="假" w389 {
          tunnel: w388 -> [w401 w412]
          tunnel: w387 -> [w404 w411]
          tunnel: [w392 w412] -> w386
          tunnel: [w403 w411] -> w385
          tunnel: w380 -> [w400 _]
          frame False {
            n131 = call "Send station config update event.vi"("error in (no error)"=w404, "Station config in"=w401) -> ("error out"=w402:errorcluster, "Station config out"=w392:refnum<class "Station config.lvclass">)  [unwired: 8 in]
            n132 = call-dynamic "Compare two recipes for differences.vi"("Baseline Recipe in"=w400, "Comparison Recipe in"=w392, "error in (no error)"=w402) -> ("Keys added"=w399:T22[], "Keys removed"=w397:T22[], "Keys with value changes"=w398:T22[], "Key change verbose details"=w393:string, "error out"=w395:errorcluster)  [unwired: 2 in, 6 out]
            n133 = Build Array (concatenate)(w399, w397, w398) -> (w396:T22[])
            n134 = Empty Array?(array=w396) -> (empty?=w394:bool)
            n135 = case shown="假" w394 {
              tunnel: [w407 w410] -> w403
              tunnel: w395 -> [w406 w410]
              tunnel: w393 -> [w405 _]
              frame False {
                n136 = call <userlib>:"Create log entry.vi"("Logging type choice"=Logging_type_choice."Station config change", "error in (no error)"=w406, "Verbose log addition (none)"=w405, "Brief log entry"="Station configuration keys changed") -> ("error out"=w407:errorcluster)  [unwired: 7 in]
              }
              frame True {
              }
            }
          }
          frame True {
          }
        }
      }
      frame "Configure instruments" {
        # "The default here is \"Super-user\" access, meaning anyone who can click the button can edit all of the setup for an instrument.  \n\nIf there is any need to control this, modify the permissions settings for this VI and/or for stored instruments setups.\n#CheckDefault"
        # "Open this type definition, and add one entry in this list for each Identifier that the station will use for its instruments.  Leaving is blank is OK if the station won't be using instruments. \n\nIf the list of instruments is not yet defined, it's best to put in a starting list of the best guesses so far and just add more or make corrections later.\n#ChangeThis"
        n137 = call-dynamic "Read Instrument setup array.vi"("error in (no error)"=w425, "Station config in"=w413) -> ("error out"=w423:errorcluster, "Instrument setup array"=w422:refnum<class "Station setup.lvclass">[], "Station config out"=w424:refnum<class "Station config.lvclass">)  [unwired: 7 in]
        n138 = call <userlib>:"Station setup user window.vi"("Is superuser? (F)"=TRUE, "Identifier list enum"=Instrument_list."" ("Instrument list"), "error in (no error)"=w423, "Station setup array in"=w422) -> ("error out"=w420:errorcluster, "Cancelled?"=w416:bool, "Station setup array out"=w421:refnum<class "Station setup.lvclass">[])  [unwired: 5 in]
        n139 = case shown="假" w416 {
          tunnel: w424 -> [w440 w448]
          tunnel: w421 -> [w426 _]
          tunnel: w420 -> [w439 w447]
          tunnel: [w437 w447] -> w417
          tunnel: [w427 w448] -> w415
          tunnel: w413 -> [w432 _]
          frame False {
            n140 = call-dynamic "Write Instrument setup array.vi"("error in (no error)"=w439, "Instrument setup array"=w426, "Station config in"=w440) -> ("error out"=w434:errorcluster, "Station config out"=w433:refnum<class "Station config.lvclass">)  [unwired: 7 in]
            n141 = call-dynamic "Compare two recipes for differences.vi"("Baseline Recipe in"=w433, "Comparison Recipe in"=w432, "error in (no error)"=w434) -> ("Baseline Recipe out"=w431:refnum<class "Station config.lvclass">, "Other recipe changes found"=w429:bool, "Other recipe changes verbose details"=w428:string, "error out"=w430:errorcluster)  [unwired: 2 in, 7 out]
            n142 = call "Send station config update event.vi"("error in (no error)"=w430, "Station config in"=w431) -> ("error out"=w438:errorcluster, "Station config out"=w427:refnum<class "Station config.lvclass">)  [unwired: 8 in]
            n143 = case shown="真" w429 {
              tunnel: w438 -> [w441 w446]
              tunnel: [w441 w445] -> w437
              tunnel: Logging_type_choice."Station config change" ("Logging type choice") -> [_ w444]
              tunnel: "Station configuration instrument setups updated" ("Brief log entry") -> [_ w443]
              tunnel: w428 -> [_ w442]
              frame False {
              }
              frame True {
                n144 = call <userlib>:"Create log entry.vi"("Logging type choice"=w444, "error in (no error)"=w446, "Verbose log addition (none)"=w442, "Brief log entry"=w443) -> ("error out"=w445:errorcluster)  [unwired: 7 in]
              }
            }
          }
          frame True {
          }
        }
      }
      frame "Upload station config" {
        # "Review all of the non-required inputs for the VI that uploads the station configuration and ensure that the defaults are OK.  \n\nIf not OK, add the changes both here and in the \"Get station configuration\" state, as many of the inputs are the same on the upload and download VIs.\n#CheckDefault"
        n145 = call-dynamic "Upload station config to MOM web interface.vi"("Station config in"=w458, "Version"="0", "Program name"=w457, "Recipe server to use? (Default production)"=Base_URI_for_MOM_recipe_management."Localhost", "Computer name override (use FQDN)"="RCX", "error in (no error)"=w459) -> ("Station config out"=w453:refnum<class "Station config.lvclass">, "Creation successful"=w452:bool, "error out"=w455:errorcluster)  [unwired: 4 in, 3 out]
        n146 = case shown="假" w452 {
          tunnel: w455 -> [w464 w467]
          tunnel: [w463 w466] -> w454
          tunnel: w453 -> [w462 _]
          frame False {
            n147 = call-dynamic "Handle any recipe problems.vi"("Recipe problem handling method"=Recipe_problem_handling_method."Check for problems, make no errors", "Pop-up messages?"=TRUE, "error in (no error)"=w464, "nLight Recipe in"=w462) -> ("error out"=w463:errorcluster)  [unwired: 4 in, 3 out]
          }
          frame True {
            n148 = One Button Dialog(message="Station config upload was successful.") -> ()  [unwired: 1 in, 1 out]
            n149 = call <userlib>:"Create log entry.vi"("Logging type choice"=Logging_type_choice."Station config change", "error in (no error)"=w467, "Brief log entry"="Station configuration uploaded") -> ("error out"=w466:errorcluster)  [unwired: 8 in]
          }
        }
      }
      frame "Edit test recipe keys" {
        # "This works the same as the key editor for the station configuration, but there are no \"starter\" enums.\n\nCreate the enums and use them if you like.\n\nAlternately, delete this entire case if you're either not using the keys at all or if you want to have all the key editing happen only in the custom manual editor window.\n#CheckDefault"
        n150 = call "Read Loaded test recipe.vi"("error in (no error)"=w476, "Fiber Auto Collimation state data in"=w471) -> ("error out"=w473:errorcluster, "Loaded test recipe"=w475:refnum<class "Test Recipe.lvclass">, "Fiber Auto Collimation state data out"=w470:refnum<class "Fiber Auto Collimation state data.lvclass">)  [unwired: 7 in]
        n151 = call <userlib>:"Key editor window.vi"("error in (no error)"=w473, "nLight Recipe in"=w475) -> ("error out"=w479:errorcluster, "Cancelled?"=w480:bool, "nLight Recipe out"=w474:refnum<class "Test Recipe.lvclass">)  [unwired: 7 in]
        n152 = case shown="假" w480 {
          tunnel: w474 -> [w482 _]
          tunnel: w479 -> [w484 w506]
          tunnel: [w493 w506] -> w478
          tunnel: w475 -> [w492 _]
          tunnel: [w483 w505] -> w472
          tunnel: w470 -> [w481 w505]
          frame False {
            n153 = call-dynamic "Compare two recipes for differences.vi"("Baseline Recipe in"=w492, "Comparison Recipe in"=w482, "error in (no error)"=w484) -> ("Keys added"=w491:T22[], "Keys removed"=w489:T22[], "Keys with value changes"=w490:T22[], "Key change verbose details"=w485:string, "error out"=w487:errorcluster)  [unwired: 2 in, 6 out]
            n154 = Build Array (concatenate)(w491, w489, w490) -> (w488:T22[])
            n155 = Empty Array?(array=w488) -> (empty?=w486:bool)
            n156 = case shown="假" w486 {
              tunnel: [w497 w504] -> w493
              tunnel: w487 -> [w500 w504]
              tunnel: w485 -> [w499 _]
              tunnel: [w496 w503] -> w483
              tunnel: w482 -> [w495 _]
              tunnel: w481 -> [w494 w503]
              frame False {
                n157 = call <userlib>:"Create log entry.vi"("Logging type choice"=Logging_type_choice."Recipe load/change", "error in (no error)"=w500, "Verbose log addition (none)"=w499, "Brief log entry"="Test recipe configuration keys changed") -> ("error out"=w498:errorcluster)  [unwired: 7 in]
                n158 = call "Write Loaded test recipe.vi"("error in (no error)"=w498, "Loaded test recipe"=w495, "Fiber Auto Collimation state data in"=w494) -> ("error out"=w497:errorcluster, "Fiber Auto Collimation state data out"=w496:refnum<class "Fiber Auto Collimation state data.lvclass">)  [unwired: 7 in]
              }
              frame True {
              }
            }
          }
          frame True {
          }
        }
      }
      frame "Edit test recipe" {
        n159 = call "Read Loaded test recipe.vi"("error in (no error)"=w516, "Fiber Auto Collimation state data in"=w515) -> ("error out"=w514:errorcluster, "Loaded test recipe"=w510:refnum<class "Test Recipe.lvclass">, "Fiber Auto Collimation state data out"=w509:refnum<class "Fiber Auto Collimation state data.lvclass">)  [unwired: 7 in]
        n160 = call-dynamic "Manual config window.vi"("error in (no error)"=w514, "nLight Recipe in"=w510) -> ("error out"=w513:errorcluster, "Cancelled?"=w512:bool, "nLight Recipe out"=w511:refnum<class "Test Recipe.lvclass">)  [unwired: 7 in]
        n161 = case shown="假" w512 {
          tunnel: w511 -> [w529 _]
          tunnel: w513 -> [w531 w538]
          tunnel: [w518 w538] -> w507
          tunnel: w510 -> [w533 _]
          tunnel: [w530 w537] -> w508
          tunnel: w509 -> [w528 w537]
          frame False {
            # "Note that the Diff VI here is only accurate if either the only changes were key changes, or if the Test Recipe was replaced with a descendant and an override was created for the \"Diff\" VI (which is highly recommended)."
            n162 = call-dynamic "Compare two recipes for differences.vi"("Baseline Recipe in"=w533, "Comparison Recipe in"=w529, "error in (no error)"=w531) -> ("Other recipe changes verbose details"=w524:string, "Key change verbose details"=w523:string, "error out"=w532:errorcluster)  [unwired: 2 in, 8 out]
            n163 = Concatenate Strings(w524, "\r\n", w523) -> (w521:string)
            n164 = call <vilib>:"Trim Whitespace.vi"("string"=w521) -> ("trimmed string"=w520:string)  [unwired: 1 in]
            n165 = call <userlib>:"Create log entry.vi"("Logging type choice"=Logging_type_choice."Recipe load/change", "error in (no error)"=w532, "Verbose log addition (none)"=w520, "Brief log entry"="Test recipe edited manually") -> ("error out"=w525:errorcluster)  [unwired: 7 in]
            n166 = call "Write Loaded test recipe.vi"("error in (no error)"=w525, "Loaded test recipe"=w529, "Fiber Auto Collimation state data in"=w528) -> ("error out"=w519:errorcluster, "Fiber Auto Collimation state data out"=w530:refnum<class "Fiber Auto Collimation state data.lvclass">)  [unwired: 7 in]
            n167 = case shown="无错误" w519 {
              selector: w519 -> [w535 w536]
              tunnel: [w535 w536] -> w518
              frame No Error {
                n168 = One Button Dialog(message="Recipe updated locally.  It is not uploaded to the recipe database.") -> ()  [unwired: 1 in, 1 out]
              }
              frame Error {
              }
            }
          }
          frame True {
          }
        }
      }
      frame "Upload test recipe" {
        n169 = call "Read Loaded test recipe.vi"("error in (no error)"=w550, "Fiber Auto Collimation state data in"=w549) -> ("error out"=w548:errorcluster, "Loaded test recipe"=w547:refnum<class "Test Recipe.lvclass">)  [unwired: 7 in, 1 out]
        n170 = call <userlib>:"Upload test recipe to MOM web interface.vi"("Recipe server to use? (Default production)"=Base_URI_for_MOM_recipe_management."Localhost", "error in (no error)"=w548, "Recipe in"=w547) -> ("error out"=w546:errorcluster, "Recipe is duplicate"=w542:bool, "RecipeID"=w543:i32, "Recipe out"=w540:refnum<class "Test Recipe.lvclass">, "Web address to view and set associations"=w541:string, "Upload worked?"=w545:bool)  [unwired: 3 in]
        n171 = case shown="假" w545 {
          tunnel: w546 -> [w556 w564]
          tunnel: [w557 w562] -> w544
          tunnel: w543 -> [_ w569]
          tunnel: w542 -> [_ w568]
          tunnel: w541 -> [_ w561]
          tunnel: w540 -> [w552 _]
          frame False {
            n172 = call-dynamic "Handle any recipe problems.vi"("Recipe problem handling method"=Recipe_problem_handling_method."Convert problems to errors", "Pop-up messages?"=FALSE, "error in (no error)"=w556, "nLight Recipe in"=w552) -> ("error out"=w555:errorcluster)  [unwired: 4 in, 3 out]
            n173 = case shown="错误" w555 {
              selector: w555 -> [w558 w560]
              tunnel: [w558 w560] -> w557
              frame No Error {
                n174 = One Button Dialog(message="Upload failed, but no error returned.") -> ()  [unwired: 1 in, 1 out]
              }
              frame Error {
              }
            }
          }
          frame True {
            n175 = Select(t=" (duplicate)", s=w568, f="") -> (s? t:f=w565:string)
            n176 = Format Into String(format string="Upload successful as recipe # %d%s.  Do you want to go to the recipe management page to set associations?" ("message"), w569, w565) -> (resulting string=w572:string)  [unwired: 2 in, 1 out]
            n177 = Two Button Dialog(message=w572, 1:"No thanks" ("F button name (\"Cancel\")"), 2:"Yes, open a browser" ("T button name (\"OK\")")) -> (T button?=w563:bool)
            n178 = case shown="真" w563 {
              tunnel: w564 -> [w574 w577]
              tunnel: [w574 w575] -> w562
              tunnel: w561 -> [_ w576]
              frame False {
              }
              frame True {
                n179 = call-poly <vilib>:"Open URL in Default Browser.vi"("error in (no error)"=w577, "URL"=w576) -> ("error out"=w575:errorcluster)  [unwired: 4 in, 1 out]
              }
            }
          }
        }
      }
      frame "Enter MOM Lot" {
        n180 = disable-structure shown="启用" {
          disable-tunnel: w584 -> [w589 w592]
          disable-tunnel: [w588 w592] -> w583
          disable-tunnel: [w587 "111" ("MOM Lot")] -> w582
          disable-tunnel: [w586 TRUE ("OK")] -> w581
          frame Disabled {
            n181 = call "MOM Lot entry"("error in (no error)"=w589) -> ("MOM Lot"=w587:string, "OK"=w586:bool, "error out"=w588:errorcluster)  [unwired: 16 in]
          }
          frame Enabled {
          }
        }
        n182 = case shown="真" w581 {
          tunnel: w583 -> [w594 w605]
          tunnel: w582 -> [_ w602]
          tunnel: [w594 w598] -> w580
          tunnel: w579 -> [w593 w603]
          tunnel: [w593 w600] -> w578
          frame False {
            # "Entry cancelled"
          }
          frame True {
            # "This is the base-level Test Recipe.  In most cases this isn't the right thing to use, and you should create a custom descendant class for this station.  The other option is to use the base class with all of the recipe data being in its keys; if you do that, make some key enums and add them to the  \"Edit test recipe keys\" case.\n\nChange this class constant (and the one in the private class data for the state data object plus its accessors) to be that new class.  If you use something else or don't use test recipes at all, remove this section (and optionally the class constant in the state data).\n#ChangeThis"
            n183 = call <userlib>:"Look up MOM lot data.vi"("MOM Lot"=w602, "error in (no error)"=w605) -> ("Lot reference out"=w597:refnum<k24>, "Lot found?"=w596:bool, "Part number"=w609:string, "Process step name"=w608:string, "Serial numbers"=w604:string[], "error out"=w607:errorcluster)  [unwired: 5 in, 3 out]
            n184 = disable-structure shown="启用" {
              disable-tunnel: w596 -> [w610 _]
              disable-tunnel: [w610 TRUE ("Lot found?")] -> w595
              frame Disabled {
              }
              frame Enabled {
                # "RCX"
              }
            }
            n185 = Array Size(array=w604) -> (size(s)=w606:i32)
            n186 = case shown="真" w595 {
              tunnel: [w614 w636] -> w599
              tunnel: w609 -> [_ _]
              tunnel: w608 -> [_ _]
              tunnel: w604 -> [_ w634]
              tunnel: w607 -> [w613 w633]
              tunnel: w606 -> [_ w635]
              tunnel: w603 -> [w612 w630]
              tunnel: w602 -> [_ w629]
              tunnel: w597 -> [_ w626]
              tunnel: refnum<class "Test Recipe.lvclass"> refnum ("Recipe model in (defaults)") -> [_ w628]
              tunnel: [w612 w627] -> w600
              frame False {
                n187 = case shown="无错误" w613 {
                  selector: w613 -> [w622 w623]
                  tunnel: [w622 w623] -> w614
                  frame No Error {
                    n188 = Unbundle(w622) -> ("source"=w620:string)  [unwired: 2 out]
                    n189 = call <vilib>:"Trim Whitespace.vi"("string"=w620) -> ("trimmed string"=w615:string)  [unwired: 1 in]
                    n190 = Empty String/Path?(string/path=w615) -> (empty?=w621:bool)
                    n191 = Concatenate Strings("ML lookup failed.  MOM says:\n\n" ("string"), w615) -> (w618:string)
                    n192 = Select(t="ML lookup failed.  MOM did not provide a reason why." ("string"), s=w621, f=w618) -> (s? t:f=w616:string)
                    n193 = One Button Dialog(message=w616) -> ()  [unwired: 1 in, 1 out]
                  }
                  frame Error {
                  }
                }
              }
              frame True {
                n194 = case shown="2.." w635 {
                  tunnel: w634 -> [_ w691 w699]
                  tunnel: w633 -> [w688 w692 w698]
                  tunnel: [w687 w692 w694] -> w632
                  tunnel: ["" w690 w693] -> w631
                  tunnel: [FALSE TRUE w696] -> w625
                  frame ..0 {
                    n195 = call <userlib>:"Insert error no loss.vi"("error message"="MOM lookup seemed to go OK but no serial numbers were found in the lot.", "error in (no error)"=w688, "error code"=8764) -> ("error out"=w687:errorcluster)  [unwired: 6 in]
                  }
                  frame 1 {
                    n196 = Index Array(array=w691) -> (element=w690:string)  [unwired: 1 in]
                  }
                  frame 2.. {
                    n197 = call <userlib>:"Choose string from array with popup.vi"("Name of thing to choose (\"item\")"="serial number" ("Name of thing to choose (\"item\")"), "error in (no error)"=w698, "Strings to choose from"=w699) -> ("error out"=w694:errorcluster, "Selection cancelled"=w695:bool, "Chosen string"=w693:string)  [unwired: 5 in, 1 out]
                    n198 = Not(x=w695) -> (.not. x?=w696:bool)
                  }
                }
                n199 = disable-structure shown="启用" {
                  disable-tunnel: w625 -> [w637 _]
                  disable-tunnel: [w637 TRUE] -> w624
                  frame Disabled {
                  }
                  frame Enabled {
                  }
                }
                n200 = case shown="真" w624 {
                  tunnel: [w640 w646] -> w636
                  tunnel: w632 -> [w640 w657]
                  tunnel: w631 -> [_ w653]
                  tunnel: w630 -> [w639 w656]
                  tunnel: w629 -> [_ w643]
                  tunnel: w626 -> [_ w652]
                  tunnel: w628 -> [_ w647]
                  tunnel: [w639 w645] -> w627
                  frame False {
                    # "SN selection cancelled, or no SNs found"
                  }
                  frame True {
                    n201 = call "Write DUT Serial.vi"("error in (no error)"=w657, "DUT Serial"=w653, "Fiber Auto Collimation state data in"=w656) -> ("error out"=w654:errorcluster, "Fiber Auto Collimation state data out"=w655:refnum<class "Fiber Auto Collimation state data.lvclass">)  [unwired: 7 in]
                    n202 = call "Write MOM Lot.vi"("error in (no error)"=w654, "MOM Lot"=w643, "Fiber Auto Collimation state data in"=w655) -> ("error out"=w651:errorcluster, "Fiber Auto Collimation state data out"=w648:refnum<class "Fiber Auto Collimation state data.lvclass">)  [unwired: 7 in]
                    n203 = call <userlib>:"Look up recipe IDs from MOM lot reference.vi"("Initialized MOM Lot in"=w652, "error in (no error)"=w651) -> ("Exactly one recipe found"=w641:bool, "Number of recipes found"=w644:i32, "Recipe ID of only recipe found"=w649:i32, "error out"=w650:errorcluster)  [unwired: 5 in, 5 out]
                    n204 = disable-structure shown="启用" {
                      disable-tunnel: [TRUE w659] -> w642
                      disable-tunnel: w641 -> [_ w659]
                      frame Enabled {
                      }
                      frame Disabled {
                      }
                    }
                    n205 = case shown="假" w642 {
                      tunnel: w650 -> [w664 w668]
                      tunnel: w649 -> [_ w675]
                      tunnel: w648 -> [w663 w682]
                      tunnel: w647 -> [_ w672]
                      tunnel: [w664 w678] -> w646
                      tunnel: [w663 w681] -> w645
                      tunnel: w644 -> [w662 _]
                      tunnel: w643 -> [_ w676]
                      frame False {
                        # "Decide what to do if something other than exactly one recipe isn't found here.  Doing nothing may be it, but usually isn't.\n#CheckDefault"
                        n206 = Format Into String(format string="MOM returned %d recipes, expected exactly 1!", w662) -> (resulting string=w661:string)  [unwired: 2 in, 1 out]
                        n207 = One Button Dialog(message=w661) -> ()  [unwired: 1 in, 1 out]
                      }
                      frame True {
                        n208 = call <userlib>:"Get MOMi common data.vi"("error in (no error)"=w668) -> ("error out"=w667:errorcluster, "Common"=w666:T24)  [unwired: 9 in]
                        n209 = call <userlib>:"Download MOM recipe by RecipeID.vi"("Recipe server to use? (Default production)"=Base_URI_for_MOM_recipe_management."Localhost", "MOMi Common"=w666, "error in (no error)"=w667, "RecipeID"=w675, "Recipe model in (defaults)"=w672) -> ("error out"=w673:errorcluster, "Actual Recipe out"=w671:refnum<class "nLight Recipe.lvclass">)  [unwired: 3 in, 2 out]
                        n210 = call "To more specific class (with better errors).vim"("Destination class type"=w672, "Class to convert"=w671, "error in (no error)"=w673) -> ("Converted class"=w670:refnum<class "Test Recipe.lvclass">, "error out"=w669:errorcluster)  [unwired: 5 in]
                        n211 = call "Write Loaded test recipe.vi"("error in (no error)"=w669, "Loaded test recipe"=w670, "Fiber Auto Collimation state data in"=w682) -> ("error out"=w679:errorcluster, "Fiber Auto Collimation state data out"=w681:refnum<class "Fiber Auto Collimation state data.lvclass">)  [unwired: 7 in]
                        n212 = Format Into String(format string="MOM lot %s loaded recipe %d", w676, w675) -> (resulting string=w674:string)  [unwired: 2 in, 1 out]
                        n213 = call <userlib>:"Create log entry.vi"("Logging type choice"=Logging_type_choice."Recipe load/change", "error in (no error)"=w679, "Brief log entry"=w674) -> ("error out"=w678:errorcluster)  [unwired: 8 in]
                      }
                    }
                  }
                }
              }
            }
            n214 = call "Short close reference with no error.vim"("reference"=w597, "error in (no error)"=w599) -> ("error out"=w598:errorcluster)  [unwired: 25 in]
          }
        }
      }
      frame "Start test" {
        # "Replace this with all of the checks that need to be done before running a test.\n\nExamples:\n* Hardware working OK\n* Serial number entered\n* MOM lot entered, and MOM says it's ready to test\n* Test recipe is valid\n\nRemember that this should only be checking information in the state data or in the variant data passed in.  Don't look at control values, local variables, etc.\n\n#ChangeThis"
        # "This is off of the main error chain ONLY because sometimes at the start of development, a LEQdb isn't set up yet.\n\nPut this back on the main error wire and remove the separate handler as soon as a LEQdb is installed and working!\n#ChangeThis"
        # "At the moment, this assumes that the entire test process will run inside of one state, the \"Run test\" state.\n\nThis might be perfectly fine, especially with many small subVIs or one big one, but splitting up the test into several different cases in the Model loop is probably best if the user needs to press any buttons on the front panel during the test that might need to insert a state.\n\nIf running in multiple states, it might be best to only enqueue one state right after another at the end of each state, instead of adding them all right at the start of the test.  That would allow for easier branching, looping, and/or cancelling.\n#CheckDefault"
        n215 = Two Button Dialog(message="Are you sure you're ready to test?\n请确认是否已正确输入MOM Lot和SN,\n并已选择要测试的SN。") -> (T button?=w700:bool)  [unwired: 2 in]
        n216 = case shown="真" w700 {
          tunnel: w706 -> [w708 w718]
          tunnel: [w707 w709] -> w705
          tunnel: [w708 w714] -> w704
          tunnel: w702 -> [w707 w715]
          tunnel: w703 -> [_ w712]
          frame False {
          }
          frame True {
            # "If this somehow fails, it just writes a zero which is OK"
            n217 = call "Enqueue many states to model loop.vi"("error in (no error)"=w715, "Enqueued states"="Collimation") -> ("error out"=w716:errorcluster)  [unwired: 7 in, 2 out]
            n218 = call "Write Test running.vi"("error in (no error)"=w716, "Test running"=TRUE, "Fiber Auto Collimation state data in"=w718) -> ("error out"=w710:errorcluster, "Fiber Auto Collimation state data out"=w711:refnum<class "Fiber Auto Collimation state data.lvclass">)  [unwired: 7 in]
            n219 = disable-structure shown="禁用" {
              disable-tunnel: [w758 w760] -> w714
              disable-tunnel: w712 -> [w755 _]
              disable-tunnel: w711 -> [w732 w760]
              disable-tunnel: w710 -> [w731 w759]
              disable-tunnel: [w726 w759] -> w709
              frame Disabled {
                # "Set to True if this is an ITAR station!\n#ChangeThis"
                # "This bit here records the test setup of the station.  In most cases it should stay; but if a station doesn't use instruments or save data at all then it can be removed.\n\nIf errors come out of this segment, then that means the LEQdb isn't set up right.  In 99% of cases that means that the LEQdb needs fixing, NOT removing or disabling this code.\n#CheckDefault"
                # "If using something other than standard laser data to save everything, replace this reference with the appropriate one, or delete it if not used at all.\n#CheckDefault"
                n220 = call "Read MOM Lot.vi"("error in (no error)"=w731, "Fiber Auto Collimation state data in"=w732) -> ("error out"=w729:errorcluster, "MOM Lot"=w721:string, "Fiber Auto Collimation state data out"=w730:refnum<class "Fiber Auto Collimation state data.lvclass">)  [unwired: 7 in]
                n221 = call "Get software version string.vi"() -> ("Software version string"=w735:string)  [unwired: 11 in]
                n222 = call-dynamic "Read Station number.vi"("Station config in"=w755) -> ("error out"=w752:errorcluster, "Station number"=w753:i32)  [unwired: 8 in, 1 out]
                n223 = call "Read DUT Serial.vi"("error in (no error)"=w729, "Fiber Auto Collimation state data in"=w730) -> ("error out"=w720:errorcluster, "DUT Serial"=w722:string, "Fiber Auto Collimation state data out"=w758:refnum<class "Fiber Auto Collimation state data.lvclass">)  [unwired: 7 in]
                n224 = Number To Decimal String(number=w753) -> (decimal integer string=w754:string)  [unwired: 1 in]
                n225 = call <userlib>:"Create new Test Setup data set.vi"("error in (no error)"=w752, "Addressing serial"=w754) -> ("error out"=w739:errorcluster, "Test Setup data out"=w737:refnum<class "Test Setup data.lvclass">)  [unwired: 8 in]
                n226 = call-dynamic "Record software version.vi"("error in (no error)"=w739, "Software version"=w735, "Test Data in"=w737) -> ("error out"=w738:errorcluster, "Test Data out"=w736:refnum<class "Test Setup data.lvclass">)  [unwired: 7 in]
                n227 = call <instrlib>:"Get instrument list.vi"("error in (no error)"=w738) -> ("error out"=w751:errorcluster, "Instrument list"=w750:refnum<class "nLight Instrument.lvclass">[])  [unwired: 9 in]
                n228 = call-dynamic "Record test setups from array of instruments.vi"("error in (no error)"=w751, "Initialized instruments array"=w750, "Test Setup data in"=w736) -> ("error out"=w749:errorcluster, "Test Setup data out"=w748:refnum<class "Test Setup data.lvclass">)  [unwired: 7 in]
                n229 = call <userlib>:"Send save and stop.vi"("error in (no error)"=w749, "Test Data in"=w748) -> ("error out"=w747:errorcluster, "Variant return data"=w746:variant)  [unwired: 6 in, 2 out]
                n230 = call "Variant to data (with better errors).vim"("type"="", "error in"=w747, "variant"=w746) -> ("error out"=w743:errorcluster, "data"=w744:string)  [unwired: 7 in]
                n231 = call <userlib>:"nLight smart error handler.vi"("error in (no error)"=w743, "Popup message if not in table (Generic message)"="Could not save Test Setup prior to running the test.  This is usually a problem with the LEQdb.  Testing will continue, but the test data will probably be lost!", "Error title if not in table [<40 chars] (\"LabVIEW error\")"="Error saving setup data" ("Error title if not in table [<40 chars] (\"LabVIEW error\")")) -> ()  [unwired: 6 in, 3 out]
                n232 = call <userlib>:"Create new Standard Laser Data set.vi"("ITAR"=FALSE, "error in (no error)"=w720, "Serial"=w722) -> ("error out"=w756:errorcluster, "Standard Laser Data reference"=w757:refnum<class "Standard Laser Data.lvclass">)  [unwired: 7 in]
                n233 = call <userlib>:"MOM Lot Number to MOM Lot ID.vi"("LotNum"=w721) -> ("error out"=w719:errorcluster, "LotID"=w728:u32)  [unwired: 8 in, 1 out]
                n234 = call-dynamic "Record test setup checksum.vi"("error in (no error)"=w756, "Test setup checksum"=w744, "Test Data in"=w757) -> ("error out"=w734:errorcluster, "Test Data out"=w733:refnum<class "Standard Laser Data.lvclass">)  [unwired: 7 in]
                n235 = call <userlib>:"Trash error.vi"("error in"=w719) -> ()  [unwired: 15 in]
                n236 = call-dynamic "Record MOM Lot ID.vi"("error in (no error)"=w734, "MOM LotID"=w728, "Standard Laser Data in"=w733) -> ("error out"=w727:errorcluster)  [unwired: 7 in, 1 out]
                n237 = Format Into String(format string="Start testing of SN %s, lot %s", w722, w721) -> (resulting string=w723:string)  [unwired: 2 in, 1 out]
                n238 = call <userlib>:"Create log entry.vi"("Logging type choice"=Logging_type_choice."Testing start/stop", "error in (no error)"=w727, "Brief log entry"=w723) -> ("error out"=w726:errorcluster)  [unwired: 8 in]
              }
              frame Enabled {
                # "RCX"
              }
            }
          }
        }
      }
      frame "Run test" {
        n239 = disable-structure shown="启用" {
          disable-tunnel: [w779 _] -> w764
          disable-tunnel: [w777 _] -> w763
          disable-tunnel: w762 -> [w775 _]
          disable-tunnel: w761 -> [w774 _]
          frame Disabled {
            # "Using this VI or a \"True\" constant wired to the \"Send any changes now\" input of a state data write accessor in the middle of a state is the \"proper\" way to update front panel indicators during the test process if they can't wait to be updated at the end of the state by default.\n\nIn this particular case, the VI here is signaling a change to test data (which is outside of the \"normal\" state data) so it couldn't have been triggered by a normal \"Send any changes now\" input."
            # "This is fake test code.  It can be run a few times to see how the state data updates are transmitted to the View loop here and in panels appropriately, but after that it should be deleted and replaced with something else.  \n\nOr, possibly deleting this whole case if \"run test\" isn't something applicable to this station.\n#ChangeThis"
            n240 = call "Read DUT Serial.vi"("error in (no error)"=w775, "Fiber Auto Collimation state data in"=w774) -> ("error out"=w772:errorcluster, "DUT Serial"=w771:string, "Fiber Auto Collimation state data out"=w773:refnum<class "Fiber Auto Collimation state data.lvclass">)  [unwired: 7 in]
            n241 = call <userlib>:"Obtain Standard Laser Data set.vi"("error in (no error)"=w772, "Serial"=w771) -> ("error out"=w770:errorcluster, "Standard Laser Data out"=w769:refnum<class "Standard Laser Data.lvclass">)  [unwired: 8 in]
            n242 = call <userlib>:"Start LIV data set.vi"("error in (no error)"=w770, "Standard Laser Data in"=w769) -> ("error out"=w767:errorcluster, "Subtest index"=w766:T25, "Standard Laser Data out"=w768:refnum<class "Standard Laser Data.lvclass">)  [unwired: 7 in]
            n243 = for {
              N: 28 -> [w810]
              shift-right: [w815] -> w780
              shift-left: w767 -> [w795]
              shift-right: [w813] -> w778
              shift-left: w773 -> [w790]
              tunnel: [w801] -> w776
              tunnel: w768 -> [w796]
              tunnel: w766 -> [w794]
              i -> [w792]
              # "This is one method of checking to see if a loop should be stopped.  It's not the only possible method;  As long as the rule that the \"Controller\" does nothing more than send messages to the \"Model\" is obeyed, it's all fine.  It could be done with a FGV, Notifier, or a channel wire to interrupt mid-case.\n\nAlternately, if the test process is spread over numerous cases that don't take too long, just cancelling by inserting a \"Cancel\" case on the front of the controller queue and having that \"Cancel\" case handle everything after that."
              n244 = Increment(x=w792) -> (x+1=w791:i32)
              n245 = Quotient & Remainder(x=w792, y=3) -> (x-y*floor(x/y)=w799:i32)  [unwired: 1 out]
              n246 = Equal?(x=2, y=w799) -> (x = y?=w797:bool)
              n247 = case shown="真" w797 {
                tunnel: w796 -> [_ w841]
                tunnel: w791 -> [_ w842]
                tunnel: w795 -> [w817 w840]
                tunnel: w794 -> [_ w835]
                tunnel: [w817 w818] -> w793
                tunnel: w790 -> [w816 w820]
                tunnel: [w816 w819] -> w789
                frame False {
                }
                frame True {
                  n248 = Random Number (0-1)() -> (number: 0 to 1=w832:dbl)
                  n249 = Add(x=w842, y=w832) -> (x+y=w830:dbl)
                  n250 = call <userlib>:"Start LIV data point.vi"("Message subtest index"=w835, "error in (no error)"=w840, "Standard Laser Data in"=w841) -> ("error out"=w839:errorcluster, "Data point index"=w834:T26, "Standard Laser Data out"=w838:refnum<class "Standard Laser Data.lvclass">)  [unwired: 6 in]
                  n251 = Increment(x=w832) -> (x+1=w831:dbl)
                  n252 = Increment(x=w830) -> (x+1=w827:dbl)
                  n253 = node(w830) -> (w837:dbl[unit])
                  n254 = Multiply(x=w827, y=w831) -> (x*y=w829:dbl)
                  n255 = call <userlib>:"Record LIV point optical power.vi"("Data point"=w834, "Subtest"=w835, "error in (no error)"=w839, "Optical power"=w837, "Standard Laser Data in"=w838) -> ("error out"=w836:errorcluster, "Standard Laser Data out"=w833:refnum<class "Standard Laser Data.lvclass">)  [unwired: 5 in]
                  n256 = node(w829) -> (w828:dbl[unit])
                  n257 = call <userlib>:"Record LIV point set current.vi"("Data point"=w834, "Subtest"=w835, "error in (no error)"=w836, "Set current"=w828, "Standard Laser Data in"=w833) -> ("error out"=w826:errorcluster, "Standard Laser Data out"=w825:refnum<class "Standard Laser Data.lvclass">)  [unwired: 5 in]
                  n258 = call-dynamic "Retrieve LIV - Last LIV data set.vi"("error in (no error)"=w826, "Standard Laser Data in"=w825) -> ("error out"=w822:errorcluster, "LIV data set"=w824:T27)  [unwired: 7 in, 1 out]
                  n259 = Unbundle By Name(w824) -> ("LIV test data"=w823:T28[])
                  n260 = for {
                    tunnel: w823 -> [w846] mode=indexing
                    tunnel: [w843] -> w821 mode=indexing
                    n261 = Unbundle By Name(w846) -> ("Set current"=w844:sgl[unit], "Optical power"=w845:sgl[unit])
                    n262 = Bundle("Set current"=w844, "Optical power"=w845) -> (w843:T29)  [unwired: 1 in]
                  }
                  n263 = call "Write LIV Test data.vi"("error in (no error)"=w822, "LIV Test data"=w821, "Fiber Auto Collimation state data in"=w820) -> ("error out"=w818:errorcluster, "Fiber Auto Collimation state data out"=w819:refnum<class "Fiber Auto Collimation state data.lvclass">)  [unwired: 7 in]
                }
              }
              n264 = Divide(x=w791, y=w810) -> (x/y=w809:dbl)
              n265 = Multiply(x=w809, y=100.0) -> (x*y=w807:dbl)
              n266 = call "Peek at model queue.vi"("error in (no error)"=w793, "Check for specific pending state (don't check)"="Cancel Test") -> ("error out"=w806:errorcluster, "Specific pending state found"=w801:bool)  [unwired: 6 in, 2 out]
              n267 = Format Into String(format string="%d%% done", w807) -> (resulting string=w812:string)  [unwired: 2 in, 1 out]
              n268 = Select(t=u32 0, s=w801, f=u32 200 ("milliseconds to wait")) -> (s? t:f=w802:u32)
              n269 = call "Write Test status.vi"("error in (no error)"=w806, "Test status"=w812, "Fiber Auto Collimation state data in"=w789) -> ("error out"=w815:errorcluster, "Fiber Auto Collimation state data out"=w814:refnum<class "Fiber Auto Collimation state data.lvclass">)  [unwired: 7 in]
              n270 = Wait (ms)(milliseconds to wait=w802) -> ()  [unwired: 1 out]
              n271 = call "Send unsent changes.vi"("Fiber Auto Collimation state data in"=w814) -> ("Fiber Auto Collimation state data out"=w813:refnum<class "Fiber Auto Collimation state data.lvclass">)  [unwired: 1 in]
            }
            n272 = case shown="真" w776 {
              tunnel: w780 -> [w786 w787]
              tunnel: [w785 w787] -> w779
              tunnel: w778 -> [w784 w788]
              tunnel: [w783 w788] -> w777
              frame False {
                # "Not cancelled"
                n273 = call "Write Test status.vi"("error in (no error)"=w786, "Test status"="Done", "Fiber Auto Collimation state data in"=w784) -> ("error out"=w785:errorcluster, "Fiber Auto Collimation state data out"=w783:refnum<class "Fiber Auto Collimation state data.lvclass">)  [unwired: 7 in]
              }
              frame True {
              }
            }
          }
          frame Enabled {
          }
        }
      }
      frame "Collimation" {
        # "自动准直"
        n274 = call "Auto Collimation Process.vi"("error in (no error)"=w851, "Fiber Auto Collimation state data in"=w848) -> ("error out"=w850:errorcluster, "Fiber Auto Collimation state data out"=w847:refnum<class "Fiber Auto Collimation state data.lvclass">)  [unwired: 8 in]
      }
      frame "Surface defect identify" {
        # "照UV前缺陷检测，只识别脏污，不识别离焦"
        n275 = call "Surface defect identify process.vi"("error in (no error)"=w855, "Fiber Auto Collimation state data in"=w853) -> ("error out"=w854:errorcluster, "Fiber Auto Collimation state data out"=w852:refnum<class "Fiber Auto Collimation state data.lvclass">)  [unwired: 8 in]
      }
      frame "Defect detection after UV" {
        # "照UV后缺陷检测，离焦识别+脏污识别"
        n276 = call "Defect detection after UV.vi"("error in (no error)"=w862, "Fiber Auto Collimation state data in"=w860, "Station config in"=w858) -> ("error out"=w861:errorcluster, "Fiber Auto Collimation state data out"=w859:refnum<class "Fiber Auto Collimation state data.lvclass">, "Station config out"=w857:refnum<class "Station config.lvclass">)  [unwired: 6 in]
      }
      frame "Signal Defect detection" {
        # "单独离焦识别"
        n277 = call "Signal Defect detection.vi"("error in (no error)"=w867, "Fiber Auto Collimation state data in"=w865) -> ("error out"=w866:errorcluster, "Fiber Auto Collimation state data out"=w864:refnum<class "Fiber Auto Collimation state data.lvclass">)  [unwired: 8 in]
      }
      frame "Save Data" {
        # "保存自动准直数据Pre-cure"
        n278 = call "Save Data Process.vi"("error in (no error)"=w873, "Fiber Auto Collimation state data in"=w871, "Station config in"=w868) -> ("error out"=w872:errorcluster, "Fiber Auto Collimation state data out"=w870:refnum<class "Fiber Auto Collimation state data.lvclass">, "Station config out"=w869:refnum<class "Station config.lvclass">)  [unwired: 6 in]
      }
      frame "End test" {
        # "It might be a good idea to do something here to prevent a user from testing again immediately without changing the serial number.  Or not, some stations might want to test several times in a row on the same part.\n#CheckDefault"
        # "This can be changed to a different class, have grading added, or removed entirely, depending on the station setup.  Should be fine if just using standard laser data, ungraded.\n#CheckDefault"
        n279 = call "Read DUT Serial.vi"("error in (no error)"=w881, "Fiber Auto Collimation state data in"=w879) -> ("error out"=w878:errorcluster, "DUT Serial"=w877:string, "Fiber Auto Collimation state data out"=w880:refnum<class "Fiber Auto Collimation state data.lvclass">)  [unwired: 7 in]
        n280 = call <userlib>:"Obtain Standard Laser Data set.vi"("error in (no error)"=w878, "Serial"=w877) -> ("error out"=w876:errorcluster, "Standard Laser Data out"=w875:refnum<class "Standard Laser Data.lvclass">)  [unwired: 8 in]
        n281 = call <userlib>:"Send save and stop.vi"("timeout in ms (60000)"=10000, "error in (no error)"=w876, "Test Data in"=w875) -> ()  [unwired: 5 in, 4 out]
        n282 = call "Write Test running.vi"("Test running"=FALSE, "Fiber Auto Collimation state data in"=w880) -> ("error out"=w884:errorcluster, "Fiber Auto Collimation state data out"=w882:refnum<class "Fiber Auto Collimation state data.lvclass">)  [unwired: 8 in]
      }
      frame "Cancel test" {
        w887 = "End test" ("Check for specific pending state (don't check)")
        # "Right now this does nothing except change the test status and enqueues ONLY the End Test state if needed if it's not already there.\n\nIf this case plus the \"End Test\" case isn't sufficient to properly cancel the test, it will need to have code added to shut down instruments safely, return things to default, save whatever test data was gathered before the test was cancelled, etc.\n\nThis to clears out any queued steps that were already enqueued before the cancellation, and that can also be changed if not desired behavior.\n#CheckDefault"
        n283 = call "Write Test status.vi"("error in (no error)"=w896, "Test status"="Cancelled", "Fiber Auto Collimation state data in"=w894) -> ("error out"=w892:errorcluster, "Fiber Auto Collimation state data out"=w895:refnum<class "Fiber Auto Collimation state data.lvclass">)  [unwired: 7 in]
        n284 = call "Peek at model queue.vi"("error in (no error)"=w892, "Check for specific pending state (don't check)"=w887) -> ("error out"=w891:errorcluster, "Specific pending state found"=w890:bool)  [unwired: 6 in, 2 out]
        n285 = case shown="假" w890 {
          tunnel: w891 -> [w900 w901]
          tunnel: w887 -> [w899 _]
          tunnel: [w898 w901] -> w889
          frame False {
            n286 = call "Enqueue one state to model.vi"("error in (no error)"=w900, "Enqueued state"=w899) -> ("error out"=w898:errorcluster)  [unwired: 9 in]
          }
          frame True {
          }
        }
        n287 = call "Selectively clear model queue.vi"("Queue clearing option"=Selective_queue_clearing_methods."Clear all that don't match", "error in (no error)"=w889, "State(s) to look for [One per line]"=w887) -> ("error out"=w888:errorcluster)  [unwired: 7 in, 1 out]
      }
      frame "Home" {
        n288 = call <instrlib>:"Get Motion Controller reference by ID.vi"("error in (no error)"=w918, "Identifier"="Thorlabs Motion") -> ("error out"=w915:errorcluster, "Motion Controller out"=w914:refnum<class "Motion Controller.lvclass">)  [unwired: 8 in]
        n289 = call-dynamic "Home axis.vi"("Wait? (T)"=TRUE, "error in (no error)"=w915, "Axis index"=T16 0, "Motion Controller in"=w914) -> ("error out"=w911:errorcluster, "Motion Controller out"=w913:refnum<class "Motion Controller.lvclass">)  [unwired: 6 in]
        n290 = call-dynamic "Measure axis position.vi"("error in (no error)"=w911, "Axis index"=T16 0, "Motion Controller in"=w913) -> ("error out"=w904:errorcluster, "Position (distance units)"=w902:dbl[unit])  [unwired: 4 in, 3 out]
        n291 = call "Write Axis Position data.vi"("error in (no error)"=w904, "Current Position"=w902, "Fiber Auto Collimation state data in"=w906) -> ("error out"=w908:errorcluster, "Fiber Auto Collimation state data out"=w907:refnum<class "Fiber Auto Collimation state data.lvclass">)  [unwired: 7 in]
        n292 = call "Write Test status.vi"("error in (no error)"=w908, "Test status"="Home Done", "Fiber Auto Collimation state data in"=w907) -> ("error out"=w903:errorcluster, "Fiber Auto Collimation state data out"=w910:refnum<class "Fiber Auto Collimation state data.lvclass">)  [unwired: 7 in]
        n293 = call "Send unsent changes.vi"("Fiber Auto Collimation state data in"=w910) -> ("Fiber Auto Collimation state data out"=w905:refnum<class "Fiber Auto Collimation state data.lvclass">)  [unwired: 1 in]
      }
      frame "Up" {
        n294 = call "Variant to data (with better errors).vim"("type"=0.0, "error in"=w932, "variant"=w930) -> ("error out"=w931:errorcluster, "data"=w928:dbl)  [unwired: 7 in]
        n295 = Absolute Value(x=w928) -> (abs(x)=w922:dbl)
        n296 = Negate(x=w922) -> (-x=w921:dbl)
        n297 = call <instrlib>:"Get Motion Controller reference by ID.vi"("error in (no error)"=w931, "Identifier"="Thorlabs Motion") -> ("error out"=w941:errorcluster, "Motion Controller out"=w940:refnum<class "Motion Controller.lvclass">)  [unwired: 8 in]
        n298 = call-poly <instrlib>:"Move axis relative polymorphic.vi"("Wait? (T)"=TRUE, "error in (no error)"=w941, "Amount to move [m] or [deg]"=w921, "Axis index"=T16 0, "Motion Controller in"=w940) -> ("error out"=w937:errorcluster, "Motion Controller out"=w939:refnum<class "Motion Controller.lvclass">)  [unwired: 5 in]
        n299 = call-dynamic "Measure axis position.vi"("error in (no error)"=w937, "Axis index"=T16 0, "Motion Controller in"=w939) -> ("error out"=w926:errorcluster, "Position (distance units)"=w924:dbl[unit])  [unwired: 4 in, 3 out]
        n300 = call "Write Axis Position data.vi"("error in (no error)"=w926, "Current Position"=w924, "Fiber Auto Collimation state data in"=w925) -> ("error out"=w927:errorcluster, "Fiber Auto Collimation state data out"=w923:refnum<class "Fiber Auto Collimation state data.lvclass">)  [unwired: 7 in]
        n301 = call "Write Test status.vi"("error in (no error)"=w927, "Test status"="Move Done", "Fiber Auto Collimation state data in"=w923) -> ("error out"=w934:errorcluster, "Fiber Auto Collimation state data out"=w936:refnum<class "Fiber Auto Collimation state data.lvclass">)  [unwired: 7 in]
        n302 = call "Send unsent changes.vi"("Fiber Auto Collimation state data in"=w936) -> ("Fiber Auto Collimation state data out"=w933:refnum<class "Fiber Auto Collimation state data.lvclass">)  [unwired: 1 in]
      }
      frame "Down" {
        n303 = call "Variant to data (with better errors).vim"("type"=0.0, "error in"=w950, "variant"=w946) -> ("error out"=w958:errorcluster, "data"=w956:dbl)  [unwired: 7 in]
        n304 = Absolute Value(x=w956) -> (abs(x)=w955:dbl)
        n305 = call <instrlib>:"Get Motion Controller reference by ID.vi"("error in (no error)"=w958, "Identifier"="Thorlabs Motion") -> ("error out"=w965:errorcluster, "Motion Controller out"=w964:refnum<class "Motion Controller.lvclass">)  [unwired: 8 in]
        n306 = call-poly <instrlib>:"Move axis relative polymorphic.vi"("Wait? (T)"=TRUE, "error in (no error)"=w965, "Amount to move [m] or [deg]"=w955, "Axis index"=T16 0, "Motion Controller in"=w964) -> ("error out"=w961:errorcluster, "Motion Controller out"=w963:refnum<class "Motion Controller.lvclass">)  [unwired: 5 in]
        n307 = call-dynamic "Measure axis position.vi"("error in (no error)"=w961, "Axis index"=T16 0, "Motion Controller in"=w963) -> ("error out"=w953:errorcluster, "Position (distance units)"=w952:dbl[unit])  [unwired: 4 in, 3 out]
        n308 = call "Write Axis Position data.vi"("error in (no error)"=w953, "Current Position"=w952, "Fiber Auto Collimation state data in"=w949) -> ("error out"=w954:errorcluster, "Fiber Auto Collimation state data out"=w951:refnum<class "Fiber Auto Collimation state data.lvclass">)  [unwired: 7 in]
        n309 = call "Write Test status.vi"("error in (no error)"=w954, "Test status"="Move Done", "Fiber Auto Collimation state data in"=w951) -> ("error out"=w947:errorcluster, "Fiber Auto Collimation state data out"=w960:refnum<class "Fiber Auto Collimation state data.lvclass">)  [unwired: 7 in]
        n310 = call "Send unsent changes.vi"("Fiber Auto Collimation state data in"=w960) -> ("Fiber Auto Collimation state data out"=w948:refnum<class "Fiber Auto Collimation state data.lvclass">)  [unwired: 1 in]
      }
      frame "Enter SN" {
        n311 = call "Variant to data (with better errors).vim"("type"="", "error in"=w977, "variant"=w975) -> ("error out"=w971:errorcluster, "data"=w972:string)  [unwired: 7 in]
        n312 = call "Write DUT Serial.vi"("error in (no error)"=w971, "DUT Serial"=w972, "Fiber Auto Collimation state data in"=w973) -> ("error out"=w970:errorcluster, "Fiber Auto Collimation state data out"=w974:refnum<class "Fiber Auto Collimation state data.lvclass">)  [unwired: 7 in]
      }
      frame "MOM Lot" {
        n313 = call "Variant to data (with better errors).vim"("type"="", "error in"=w985, "variant"=w984) -> ("error out"=w983:errorcluster, "data"=w982:string)  [unwired: 7 in]
        n314 = call "Write MOM Lot.vi"("error in (no error)"=w983, "MOM Lot"=w982, "Fiber Auto Collimation state data in"=w981) -> ("error out"=w979:errorcluster, "Fiber Auto Collimation state data out"=w980:refnum<class "Fiber Auto Collimation state data.lvclass">)  [unwired: 7 in]
      }
      frame "Enter Fiber Ass PN" {
        n315 = call "Variant to data (with better errors).vim"("type"="", "error in"=w994, "variant"=w993) -> ("error out"=w992:errorcluster, "data"=w991:string)  [unwired: 7 in]
        n316 = call "Write Fiber Ass PN.vi"("error in (no error)"=w992, "Fiber Ass PN"=w991, "Fiber Auto Collimation state data in"=w990) -> ("error out"=w988:errorcluster, "Fiber Auto Collimation state data out"=w989:refnum<class "Fiber Auto Collimation state data.lvclass">)  [unwired: 7 in]
      }
      frame "Enter Operator" {
        n317 = call "Variant to data (with better errors).vim"("type"="", "error in"=w1002, "variant"=w1003) -> ("error out"=w1001:errorcluster, "data"=w998:string)  [unwired: 7 in]
        n318 = call "Write Operator.vi"("error in (no error)"=w1001, "Operator"=w998, "Fiber Auto Collimation state data in"=w1000) -> ("error out"=w997:errorcluster, "Fiber Auto Collimation state data out"=w999:refnum<class "Fiber Auto Collimation state data.lvclass">)  [unwired: 7 in]
      }
    }
    n319 = Or(x=w54, y=w52) -> (x .or. y?=w53:bool)
    n320 = call "Send unsent changes.vi"("Fiber Auto Collimation state data in"=w44) -> ("Fiber Auto Collimation state data out"=w43:refnum<class "Fiber Auto Collimation state data.lvclass">)  [unwired: 1 in]
    n321 = call "Apex model error handler.vi"("Next state if error"=w51, "Error codes to ignore (none)"=w42, "Current state"=w50, "error in (no error)"=w55) -> ("error out"=w49:errorcluster)  [unwired: 7 in]
  }
  n322 = while {
    tunnel: [w1015] -> w3
    shift-right: [w1011] -> _
    shift-left: _ -> [w1010]
    shift-right: [w1009] -> _
    shift-left: w11 -> [w1014]
    shift-right: [w1008] -> _
    shift-left: _ -> [w1007]
    tunnel: w1 -> [w1006]
    stop <- w1012 stop-if-true
    # "View loop.  All writes to controls go here.  Property nodes go here, but only one per control.  Write-only local variables allowed for controls.  Not allowed: global variables, enqueueing states in Model loop, instrument communication, delays."
    n323 = event "View" shown="[3] <事件注册引用句柄.Update Control(s)>: 用户事件" {
      selector: w1014 -> [_ _ _ w1084]
      dyn-events: [_ _ _ w1077] -> w1009
      timeout: _ -> [_ _ _ _]
      tunnel: [_ w1020 w1027 w1066] -> w1013
      tunnel: [TRUE _ _ _] -> w1012
      tunnel: [w1017 w1024 w1028 w1067] -> w1011
      tunnel: w1010 -> [w1017 w1024 _ w1067]
      tunnel: [w1016 w1023 w1026 w1064] -> w1008
      tunnel: w1007 -> [w1016 _ w1026 w1064]
      tunnel: w1006 -> [_ w1019 w1025 w1063]
      event User Event {
        n324 = event-data() -> ()  [unwired: 1 in, 1 out]
      }
      event User Event {
        # "This case should be called once at the start after the configuration is downloaded, and after that only very rarely, if someone changes the configuration."
        n325 = event-data() -> ("Update Station config"=w1023:refnum<class "Station config.lvclass">)  [unwired: 1 in]
        n326 = control-ref of="Station information"() -> (w1022:refnum<vi>)
        n327 = call "Send update control(s) event.vim"("Fiber Auto Collimation panel"=w1019, "Control(s) [String or reference, can be array]"=w1022) -> ("error out"=w1021:errorcluster)  [unwired: 9 in]
        n328 = Build Array(w1021) -> (w1020:errorcluster[])
      }
      event User Event {
        # "All indicators should be in the case that controls their use.  That will be in this event frame if it is a \"super simple\" case, or in the \"Update control(s)\" event frame if it is more complex."
        # "This is here for easy copy-pasting, since it's used in quite a lot of new cases created to the right.  It can be removed if desired."
        # "Note that any state data that isn't displayed on this particular panel (or affects any control's appearance) should just not have a case made for it.  \n\nDoing nothing in the Default case takes care of it, and if it needs to be displayed or checked later a case can be added then."
        # "For each case here there should be EXACTLY ONE of two things happening:\n\n1. (Super simple case) The read accessor for one piece of state data writes to one indicator terminal (not a local variable! No property nodes!), and nothing else.\n2. (Anything else) A list of any and all controls that could be affected by a change in this state data is sent to the \"Send update control(s) event.vim\", and nothing else.\n\nFor the \"Anything else\" situation, note that \"Send update control(s) event.vim\" is malleable and as such, can take as input a string, an array of strings, a reference to a control, or an array of control references."
        n329 = event-data() -> ("Update state data"=w1028:refnum<class "Fiber Auto Collimation state data.lvclass">)  [unwired: 1 in]
        n330 = disable-structure shown="Disabled" {
          frame Disabled {
            n331 = call "Send update control(s) event.vim"() -> ()  [unwired: 11 in, 1 out]
          }
          frame Enabled {
          }
        }
        n332 = call "Read Changed data list.vi"("Fiber Auto Collimation state data in"=w1028) -> ("error out"=w1030:errorcluster, "Changed data list"=w1031:T11[], "Fiber Auto Collimation state data out"=w1029:refnum<class "Fiber Auto Collimation state data.lvclass">)  [unwired: 8 in]
        n333 = for {
          tunnel: w1031 -> [w1036] mode=indexing
          tunnel: w1029 -> [w1035]
          tunnel: w1030 -> [w1034]
          tunnel: [w1033] -> w1027 mode=indexing
          tunnel: w1025 -> [w1032]
          n334 = case shown="\"Station status\"" w1036 {
            selector: w1036 -> [w1038 _ _ _ _]
            tunnel: w1035 -> [_ w1047 w1049 w1055 _]
            tunnel: w1034 -> [w1040 w1048 w1052 w1056 w1062]
            tunnel: [w1039 w1046 w1051 w1053 w1059] -> w1033
            tunnel: w1032 -> [_ _ _ _ w1058]
            frame Default {
              w1037 = TRUE  # Ignore errors from this case?
              # "This defaults to True because a lot of state data doesn't immediately get displayed on a control on the front panel.\n\nChange this to False if you want to get errors about state data updating that doesn't have a case here to display it.\n#CheckDefault"
              n335 = case shown="假" w1037 {
                tunnel: w1040 -> [w1043 w1044]
                tunnel: [w1042 w1044] -> w1039
                tunnel: w1038 -> [w1041 _]
                frame False {
                  n336 = call <userlib>:"Insert not implemented error.vi"("error in (no error)"=w1043, "Name or enum of feature not implemented (no name)"=w1041) -> ("error out"=w1042:errorcluster)  [unwired: 9 in]
                }
                frame True {
                }
              }
            }
            frame "Permission level" {
              n337 = call "Read Permission level.vi"("error in (no error)"=w1048, "Fiber Auto Collimation state data in"=w1047) -> ("error out"=w1046:errorcluster, "Permission level"=→"Permission level":T1)  [unwired: 7 in, 1 out]
            }
            frame "Username" {
              n338 = call "Read Username.vi"("error in (no error)"=w1052, "Fiber Auto Collimation state data in"=w1049) -> ("error out"=w1051:errorcluster, "Username"=→"Username":string)  [unwired: 7 in, 1 out]
            }
            frame "Model case running" {
              n339 = call "Read Model case running.vi"("error in (no error)"=w1056, "Fiber Auto Collimation state data in"=w1055) -> ("error out"=w1053:errorcluster, "Model case running"=→"Currently running state":string)  [unwired: 5 in, 3 out]
            }
            frame "Station status" {
              # "Note that this isn't a \"control\", but that's OK.  Anything passed into the \"send update\" VI just has to have a matching case in the \"update controls\" event case, whether or not it's an actual control.  \n\nIn this case, it's a signal that the appearance of this VI's front panel may need to change."
              n340 = call "Send update control(s) event.vim"("Fiber Auto Collimation panel"=w1058, "error in"=w1062, "Control(s) [String or reference, can be array]"="Front panel") -> ("error out"=w1060:errorcluster)  [unwired: 8 in]
              n341 = control-ref of="Station status"() -> (w1057:refnum<vi>)
              n342 = call "Send update control(s) event.vim"("Fiber Auto Collimation panel"=w1058, "error in"=w1060, "Control(s) [String or reference, can be array]"=w1057) -> ("error out"=w1059:errorcluster)  [unwired: 8 in]
            }
          }
        }
      }
      event User Event {
        # "All indicator terminals should be in the case here that controls their value and appearance.\n\nControl terminals should only be here in the rare case that they don't have any events in the Controller loop."
        # "These bits at the bottom here defer panel updating until all controls that needed to be updated have been.  Property nodes of controls take a nontrivial amount of time unless updating is deferred."
        # "This bit at the top destroys its own event registration and then recreates it.  What this actually ends up doing is killing all pending events of this type while leaving all other pending events intact.  This is because this case runs off a stored list of jobs to do (to prevent duplicates) and not its actual event data.  Since it should only ever be sent by this exact View loop to this exact View loop, there's no chance an event will get missed in the microsecond between the destruction and re-registration."
        n343 = event-data() -> ()  [unwired: 1 in, 1 out]
        n344 = Unbundle(w1084) -> ("事件注册引用句柄"=w1082:refnum<event-registration>, "事件注册引用句柄"=w1083:refnum<event-registration>)
        n345 = property class="VI"() -> (error out=w1076:errorcluster, "Panel"=w1074:refnum<vi>)  [unwired: 2 in, 1 out]
        n346 = call "Dequeue all update control strings, remove duplicates.vi"("Fiber Auto Collimation panel"=w1063) -> ("error out"=w1071:errorcluster, "Controls to update"=w1070:string[])  [unwired: 9 in]
        n347 = Unregister For Events(event registration refnum=w1082) -> (error out=w1081:errorcluster)  [unwired: 1 in]
        n348 = call "Obtain update control(s) event.vi"("error in (no error)"=w1081, "Fiber Auto Collimation panel"=w1063) -> ("error out"=w1080:errorcluster, "Update Control(s)"=w1079:refnum<user-event>)  [unwired: 8 in]
        n349 = property class="Pnl"(reference=w1074, error in=w1076, "DeferPanUpdts"=TRUE ("Defer Panel Updates")) -> (reference out=w1072:refnum<vi>, error out=w1069:errorcluster)
        n350 = register-events(error in=w1080, w1079) -> (reference out=w1078:refnum<event-registration>, error out=w1065:errorcluster)  [unwired: 1 in]
        n351 = for {
          tunnel: w1071 -> [w1089]
          tunnel: w1070 -> [w1090] mode=indexing
          tunnel: [w1088] -> w1066 mode=indexing
          tunnel: w1069 -> [w1087]
          tunnel: [w1087] -> w1068
          tunnel: w1067 -> [w1086]
          tunnel: w1065 -> [_]
          tunnel: w1064 -> [w1085]
          n352 = case shown="\"Station information\"" w1090 {
            selector: w1090 -> [w1093 _ _ _]
            tunnel: w1089 -> [w1092 w1105 w1110 w1114]
            tunnel: [w1091 w1104 w1108 w1112] -> w1088
            tunnel: w1086 -> [_ w1102 w1109 _]
            tunnel: w1085 -> [_ _ _ w1111]
            frame Default {
              n353 = Format Into String(format string="Default case reached in \"Update control(s)\" event!\nIntended control name was \"%s\".", w1093) -> (resulting string=w1094:string)  [unwired: 2 in, 1 out]
              n354 = call <userlib>:"Insert impossible case error.vi"("error in (no error)"=w1092, "Optional extra info"=w1094) -> ("error out"=w1091:errorcluster)  [unwired: 9 in]
            }
            frame "Front panel" {
              # "#TODO Set this to close/hide the panel when station is \"running\""
              # "Note that this isn't a \"control\", but that's OK.  It's allowed to have special cases here as long as they still fit the model.  In this case, it's the appearance of the front panel of this VI."
              n355 = call "Read Station status.vi"("error in (no error)"=w1105, "Fiber Auto Collimation state data in"=w1102) -> ("error out"=w1103:errorcluster, "Station status"=w1101:T3)  [unwired: 7 in, 1 out]
              n356 = Equal?(x=w1101, y=Station_status."Running") -> (x = y?=w1099:bool)
              n357 = Select(t=T30."Hidden" ("State"), s=w1099, f=T30."Standard" ("State")) -> (s? t:f=w1096:T30)
              n358 = invoke class="VI" method="FP.Open"(error in=w1103, "State"=w1096) -> (error out=w1104:errorcluster)  [unwired: 3 in, 4 out]
            }
            frame "Station status" {
              n359 = call "Read Station status.vi"("error in (no error)"=w1110, "Fiber Auto Collimation state data in"=w1109) -> ("error out"=w1108:errorcluster, "Station status"=w1107:T3)  [unwired: 7 in, 1 out]
              n360 = Format Into String(w1107) -> (resulting string=→"Station status":string)  [unwired: 3 in, 1 out]
            }
            frame "Station information" {
              w1128 = FALSE ("Error on not found (T)")
              # "The \"software version\" field should be displayed somewhere in nearly all cases.  If it's removed from here, it needs to be made accessible elsewhere (for instance, in a \"Help->About\" menu option).\n\nThe other fields displayed in the default readout may be removed if considered unnecessary or confusing for a given station, or extra fields added.\n#CheckDefault"
              n361 = call <userlib>:"Look up string key.vi"("Error on not found (T)"=w1128, "Key [string/enum]"=String_keys."Software name" ("Station config string keys"), "error in (no error)"=w1114, "nLight Recipe in"=w1111) -> ("error out"=w1130:errorcluster, "String Key Value"=w1132:string, "nLight Recipe out"=w1131:refnum<class "Station config.lvclass">)  [unwired: 4 in, 1 out]
              n362 = call <userlib>:"Look up string key.vi"("Error on not found (T)"=w1128, "Key [string/enum]"=String_keys."Software version" ("Station config string keys"), "error in (no error)"=w1130, "nLight Recipe in"=w1131) -> ("error out"=w1125:errorcluster, "String Key Value"=w1127:string, "nLight Recipe out"=w1126:refnum<class "Station config.lvclass">)  [unwired: 4 in, 1 out]
              n363 = call <userlib>:"Read Site.vi"("error in (no error)"=w1125, "Station config in"=w1126) -> ("error out"=w1123:errorcluster, "Site"=w1115:T31, "Station config out"=w1124:refnum<class "Station config.lvclass">)  [unwired: 7 in]
              n364 = call <userlib>:"Read Environment.vi"("error in (no error)"=w1123, "Station config in"=w1124) -> ("error out"=w1121:errorcluster, "Environment"=w1116:T32, "Station config out"=w1122:refnum<class "Station config.lvclass">)  [unwired: 7 in]
              n365 = call-dynamic "Read Station number.vi"("error in (no error)"=w1121, "Station config in"=w1122) -> ("error out"=w1119:errorcluster, "Station number"=w1117:i32, "Station config out"=w1120:refnum<class "Station config.lvclass">)  [unwired: 7 in]
              n366 = call <userlib>:"Read Equipment ID.vi"("error in (no error)"=w1119, "Station config in"=w1120) -> ("error out"=w1112:errorcluster, "Equipment ID"=w1118:string)  [unwired: 7 in, 1 out]
              n367 = Format Into String(format string="Software name: %s\nSoftware version: %s\nSite: %s\nEnvironment: %s\nNEQdb Station number: %d\nMOM Equipment ID: %s", w1132, w1127, w1115, w1116, w1117, w1118) -> (resulting string=→"Station information":string)  [unwired: 2 in, 1 out]
            }
          }
        }
        n368 = Bundle("事件注册引用句柄"=w1078, "事件注册引用句柄"=w1083) -> (w1077:T2)  [unwired: 1 in]
        n369 = property class="Pnl"(reference=w1072, error in=w1068, "DeferPanUpdts"=FALSE ("Defer Panel Updates")) -> ()  [unwired: 2 out]
      }
    }
    n370 = call "Apex view loop error handler.vi"("errors in"=w1013) -> ("error out"=w1015:errorcluster)  [unwired: 10 in]
  }
  n371 = while {
    tunnel: [w1139] -> w4
    tunnel: w20 -> [w1138]
    tunnel: w14 -> [w1135]
    stop <- w1137 stop-if-true
    # "For easy copying"
    # "Controller loop.  All \"value change\" events, and any triggered by user action (menus, keys, mouse clicks, etc.).  Most event states should do nothing except enqueue to the Model loop.\nValues from associated controls should be sent to the Model in the Variant data, so reading from local variables and property nodes is allowed.  Not allowed: writing to indicators, property nodes, local variables, or global variables.  No invoke nodes."
    n372 = event "Controller [Value change events go here]" shown="[2] \"Upload station config\": 值改变" {
      selector: w1138 -> [_ _ _ _ _ _]
      dyn-events: _ -> [_ _ _ _ _ _]
      timeout: _ -> [_ _ _ _ _ _]
      tunnel: [TRUE _ _ _ _ _] -> w1137
      tunnel: [w1140 w1144 w1153 w1154 w1156 w1158] -> w1136
      tunnel: w1135 -> [_ w1148 _ _ _ _]
      event User Event {
        n373 = event-data() -> ()  [unwired: 1 in, 5 out]
        n374 = call <vilib>:"Clear Errors.vi"() -> ("error out"=w1140:errorcluster)  [unwired: 6 in, 1 out]
      }
      event Panel Close? {
        # "This window will be hidden or busy most of the time, except when there are problems getting the station confuration.  So during the times that it's shown, this is an allowable button press."
        # "If this was live LabVIEW, we always want the window to stay open. during runtime.\nIf this was an EXE, the window only closes after all the program is done, at which point the \"Exit\" call closes it.\nSo we always want to discard this here."
        # "If a \"Quit\" button or menu option is added in addition to this event (which fires when the \"X\" to close is clicked), then make sure both cases run the same code.\n\nIf there are conditions that should prevent the \"quit\" case from running (for instance, by default it's not allowed to quit during a test), instead of checking for them here or in the Model loop \"Quit\" case, it might be better to have the \"View\" loop set the \"FP.Closeable\" property of the main VI to False, and disabling any other menu item or button that also attempts to quit.  \n#CheckDefault"
        n375 = event-data() -> ()  [unwired: 1 in, 4 out]
        n376 = Format Into String(format string="Are you sure you want to exit %s?" ("message"), w1148) -> (resulting string=w1147:string)  [unwired: 2 in, 1 out]
        n377 = Two Button Dialog(message=w1147, 1:"Cancel" ("F button name (\"Cancel\")"), 2:"Yes, exit" ("T button name (\"OK\")")) -> (T button?=w1143:bool)
        n378 = case shown="真" w1143 {
          tunnel: [_ w1151] -> w1144
          frame False {
          }
          frame True {
            n379 = call "Enqueue one state to model.vi"("Enqueued state"="Quit") -> ("error out"=w1151:errorcluster)  [unwired: 10 in]
          }
        }
        n380 = event-data("Discard?"=TRUE) -> ()  [unwired: 1 in, 1 out]
      }
      event "Upload station config": Value Change {
        n381 = event-data() -> ()  [unwired: 1 in, 6 out]
        n382 = call "Enqueue one state to model.vi"("Enqueued state"="Upload station config") -> ("error out"=w1153:errorcluster)  [unwired: 10 in]
      }
      event "Configure instruments": Value Change {
        n383 = event-data() -> ()  [unwired: 1 in, 6 out]
        n384 = call "Enqueue one state to model.vi"("Enqueued state"="Configure instruments") -> ("error out"=w1154:errorcluster)  [unwired: 10 in]
      }
      event "Edit station config keys": Value Change {
        n385 = event-data() -> ()  [unwired: 1 in, 6 out]
        n386 = call "Enqueue one state to model.vi"("Enqueued state"="Edit station config keys") -> ("error out"=w1156:errorcluster)  [unwired: 10 in]
      }
      event "Basic station config": Value Change {
        n387 = event-data() -> ()  [unwired: 1 in, 6 out]
        n388 = call "Enqueue one state to model.vi"("Enqueued state"="Basic station config") -> ("error out"=w1158:errorcluster)  [unwired: 10 in]
      }
    }
    n389 = disable-structure shown="Disabled" {
      frame Disabled {
        n390 = call "Enqueue one state to model.vi"() -> ()  [unwired: 11 in, 1 out]
      }
      frame Enabled {
      }
    }
    n391 = call "Apex controller loop error handler.vi"("error in"=w1136) -> ("error out"=w1139:errorcluster)  [unwired: 10 in]
  }
  n392 = control-ref of="This VI"() -> (w2:refnum<vi>)
  n393 = call "Emergency kill loop by reference.vi"("VI reference in"=w2) -> ("error out"=w24:errorcluster)  [unwired: 10 in]
  n394 = call <userlib>:"nLight smart error handler.vi"("error in (no error)"=w38, "Error title if not in table [<40 chars] (\"LabVIEW error\")"="Error stopping station" ("Title [~40 chars max] (\"LabVIEW error\")")) -> ("error out"=w36:errorcluster)  [unwired: 7 in, 2 out]
  n395 = call <vilib>:"Clear Errors.vi"("error in (no error)"=w36) -> ("error out"=w35:errorcluster)  [unwired: 5 in, 1 out]
  n396 = call "Obtain shut down event.vi"("error in (no error)"=w35) -> ("error out"=w34:errorcluster, "Shut down"=w33:refnum<user-event>)  [unwired: 9 in]
  n397 = Generate User Event(user event=w33, event data cluster=FALSE ("event data"), error in=w34) -> (user event out=w28:refnum<user-event>, error out=w31:errorcluster)  [unwired: 1 in]
  n398 = call <userlib>:"Merge errors no loss micro.vi"("error in (no error) 1"=w31, "error in (no error) 5"=w3, "error in (no error) 7"=w4) -> ("error out"=w29:errorcluster)  [unwired: 6 in]
  n399 = call <vilib>:"Clear Errors.vi"("error in (no error)"=w29) -> ("error out"=w30:errorcluster)  [unwired: 5 in, 1 out]
  n400 = Generate User Event(user event=w28, event data cluster=TRUE ("event data"), error in=w30) -> (error out=w26:errorcluster)  [unwired: 1 in, 1 out]
  n401 = call <userlib>:"Merge errors no loss micro.vi"("error in (no error) 1"=w26, "error in (no error) 6"=w24) -> ("error out"=w25:errorcluster)  [unwired: 7 in]
  n402 = call <userlib>:"Exit if compiled into EXE.vi"("error in (no error)"=w25) -> ()  [unwired: 11 in]
